vi "PiecesMovement.vi"(8 "Move to":i32[](array[numeric]), 9 "Move from":i32[](array[numeric]), 10 "Turn":T1, 11 "Input Squares":T2[][](array[typedef])) -> (0 "Short Castle?":bool, 1 "Beat in the Passage?":bool, 2 "Last Square?":bool, 3 "Possible Move?":bool, 4 "Long Castle?":bool, 5 "Possible Moves":bool[][](array[boolean]))   [LabVIEW 2019]
doc: "This VI checks if movement of the piece is executed properly"
uses:
  #typedef_SquareType.ctl
  #typedef_Color.ctl
  #typedef_Piece.ctl
  #typedef_PieceType.ctl
panel:
  out "?":u16[][](array[ring])
  out "Last Square":bool[][](array[boolean])
  out "Beat in the Passage":bool[][](array[boolean])
  out "Short Castle":bool[][](array[boolean])
  out "Long Castle":bool[][](array[boolean])
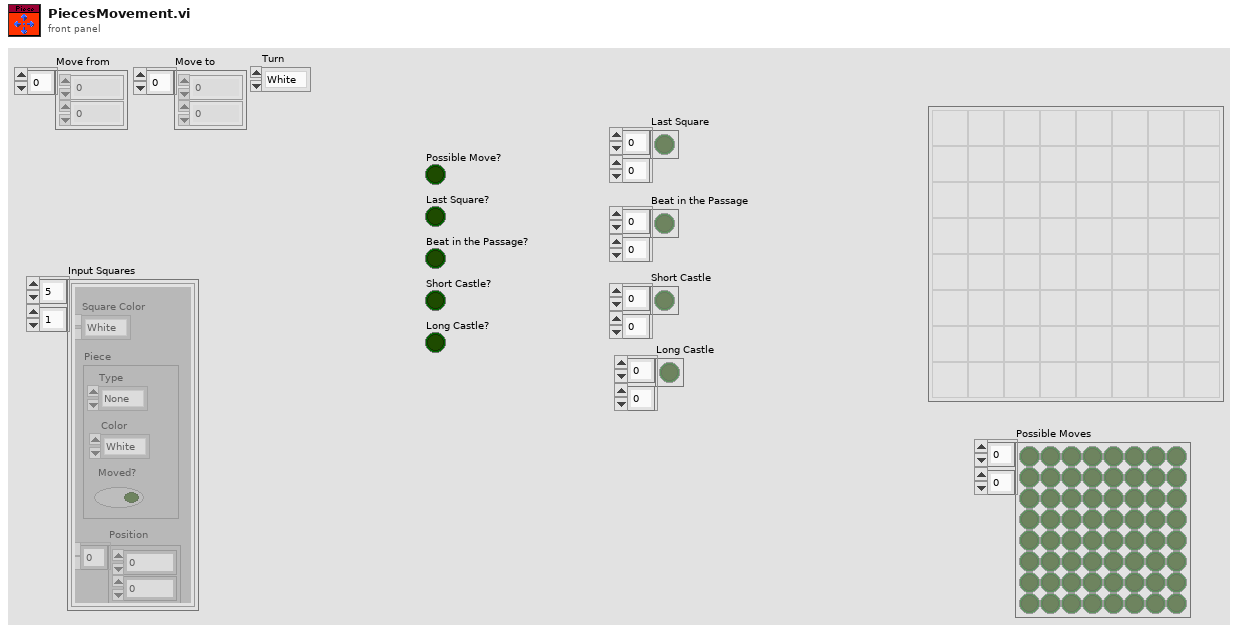
[diagram p1: front panel]
types:
  T1 = typedef "#typedef_Color.ctl" = enum16{"White", "Black"}
  T2 = typedef "#typedef_SquareType.ctl" = cluster{"Square Color":T1, "Position":i32[], "Piece":T3}
  T3 = typedef "#typedef_Piece.ctl" = cluster{"Type":T4, "Color":T1, "Moved?":bool}
  T4 = typedef "#typedef_PieceType.ctl" = enum16{"None", "Pawn", "Knight", "Bishop", "Rook", "Queen", "King"}
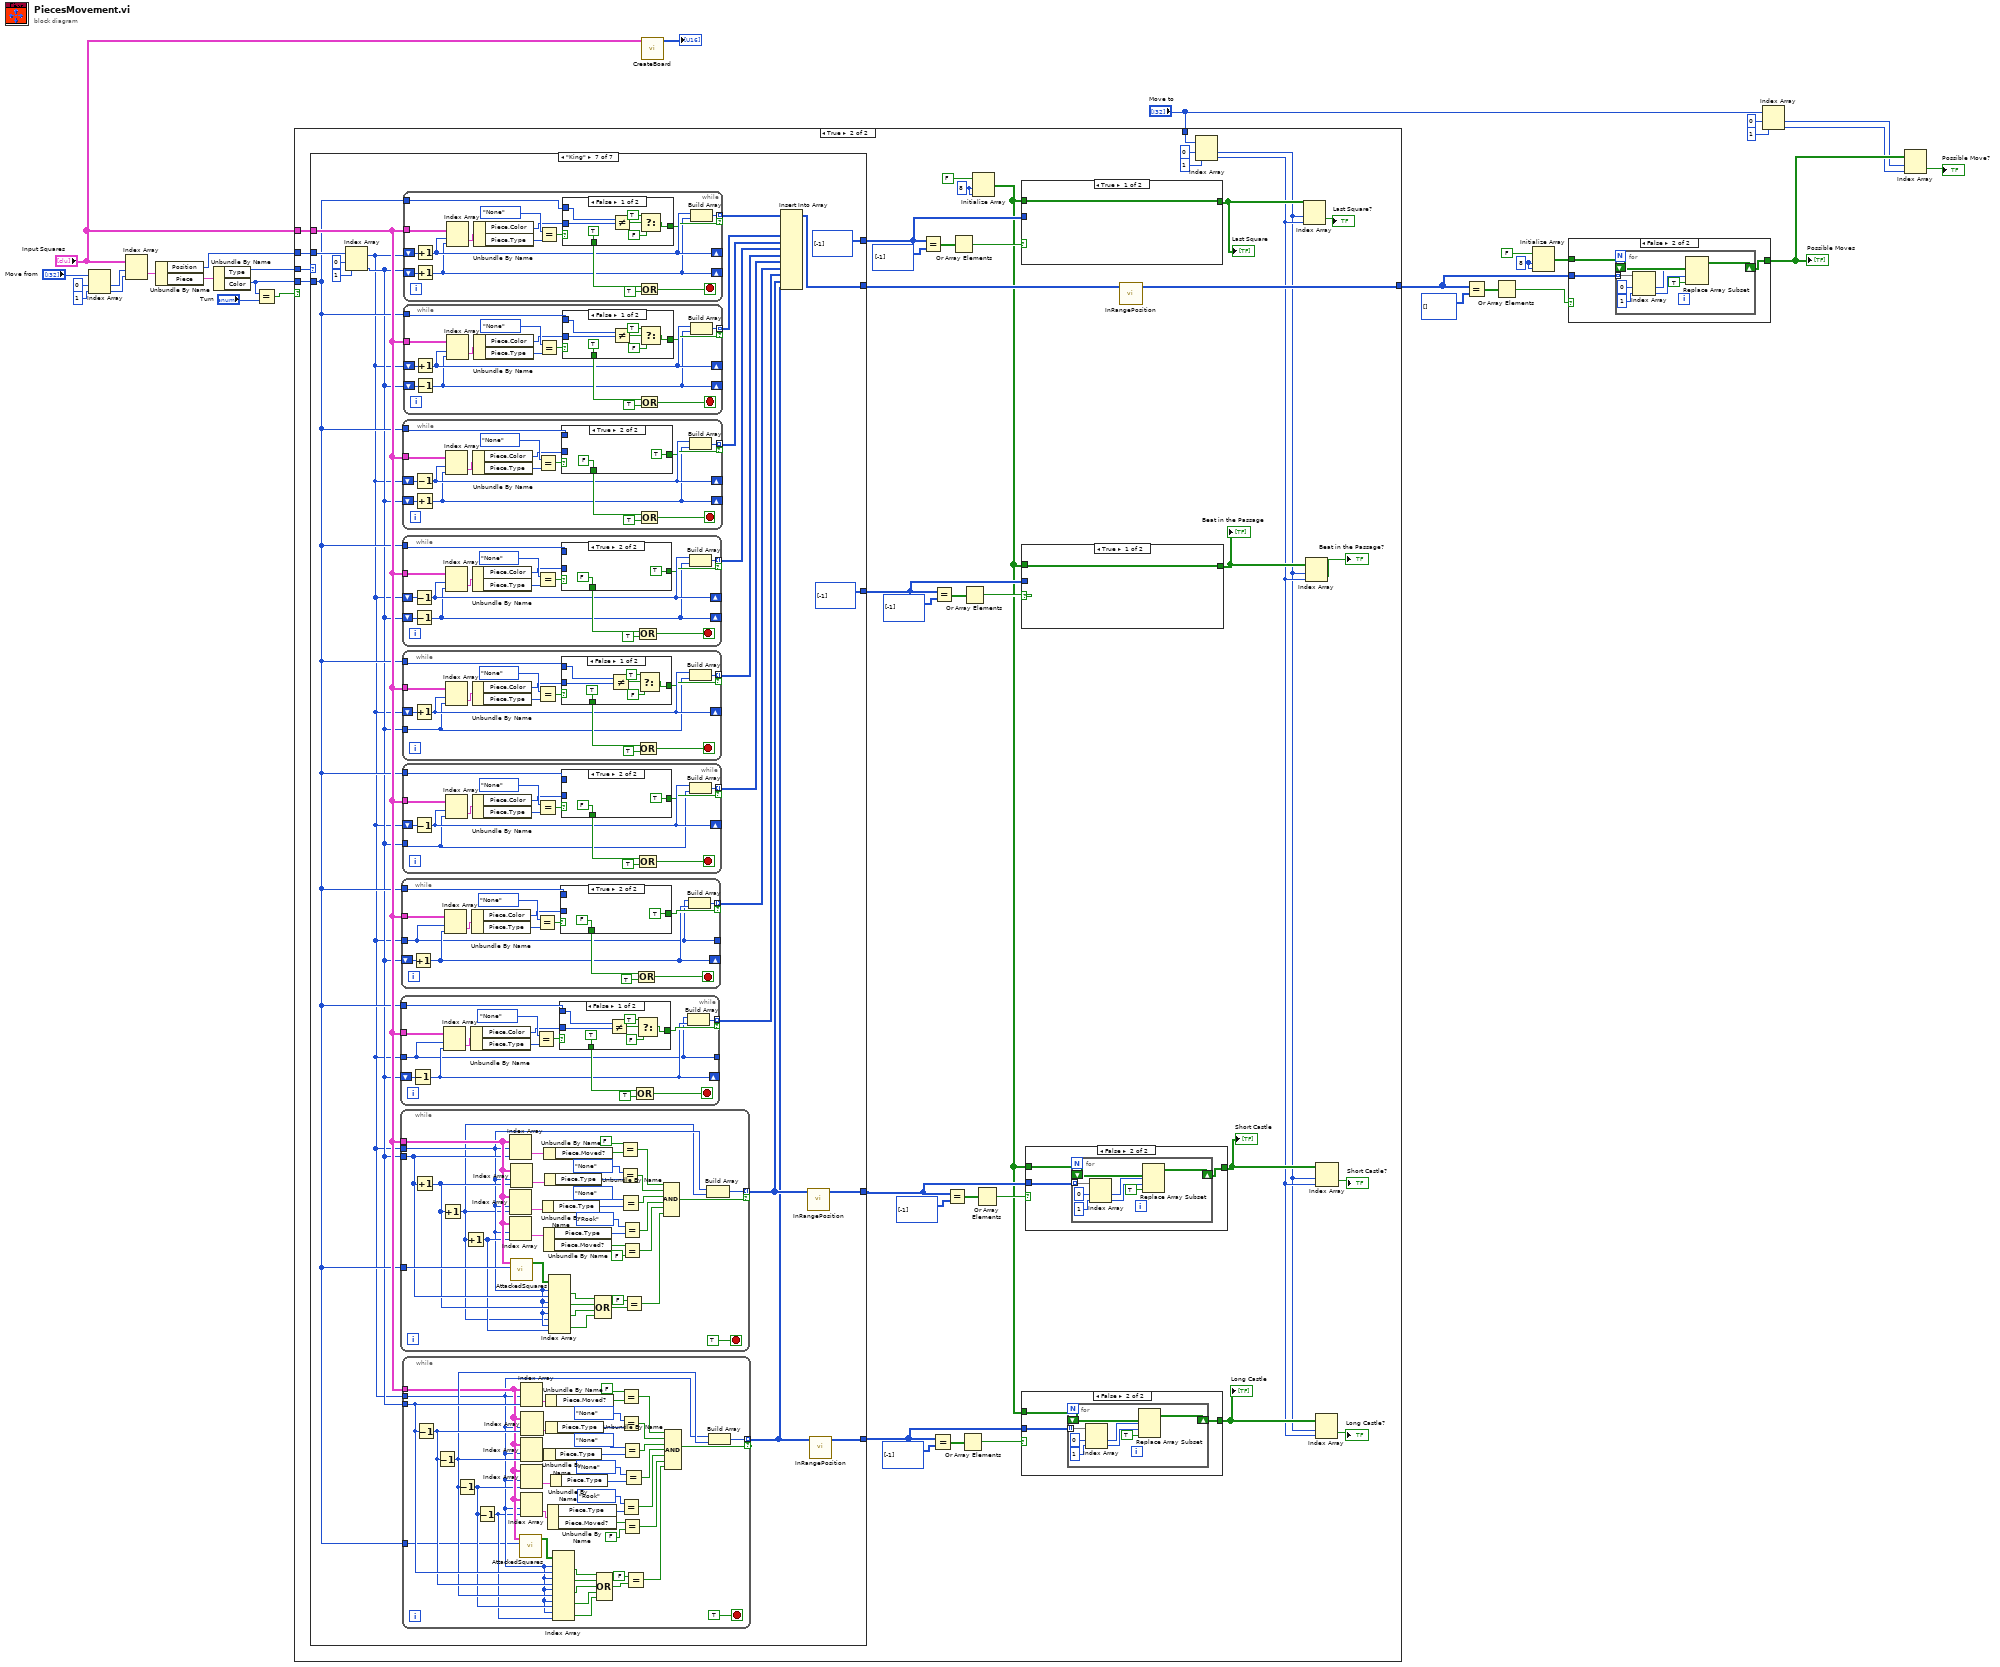
[diagram p0: block diagram]
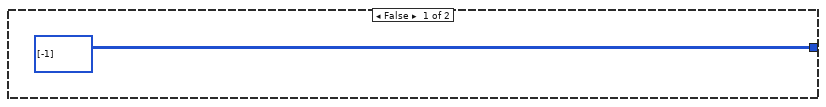
[diagram p3: hidden frame]
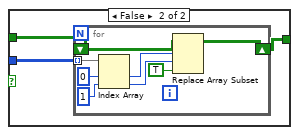
[diagram p6: hidden frame]
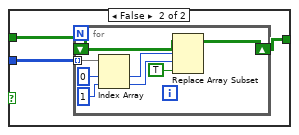
[diagram p7: hidden frame]
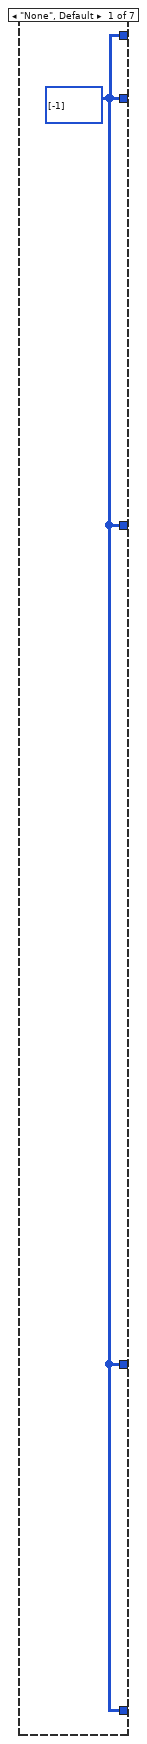
[diagram p8: hidden frame]
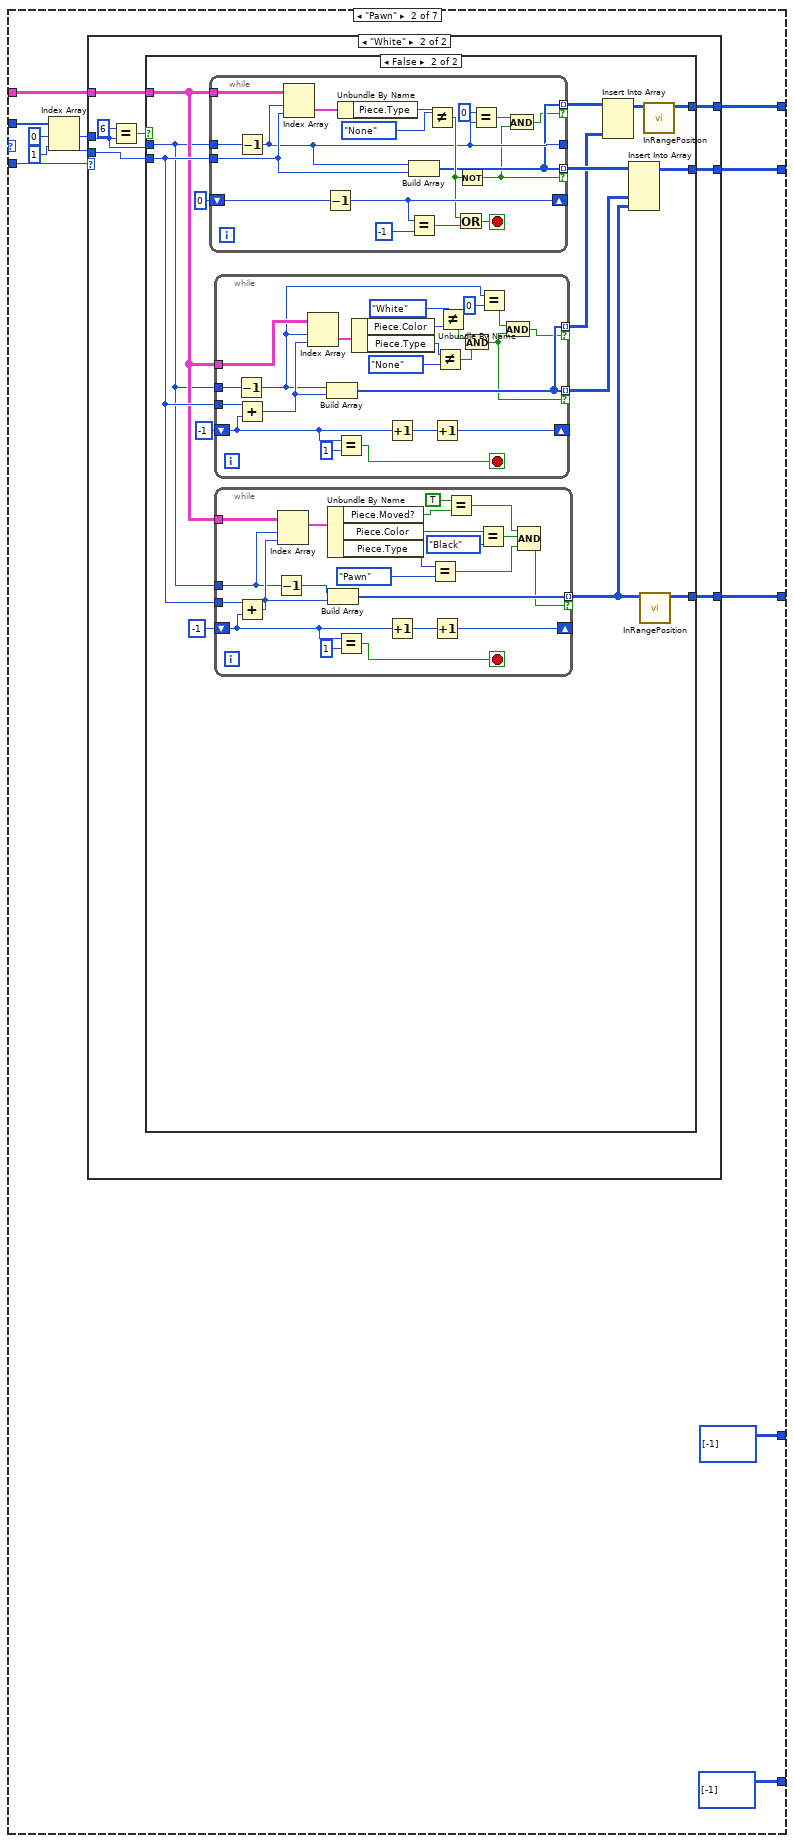
[diagram p9: hidden frame]
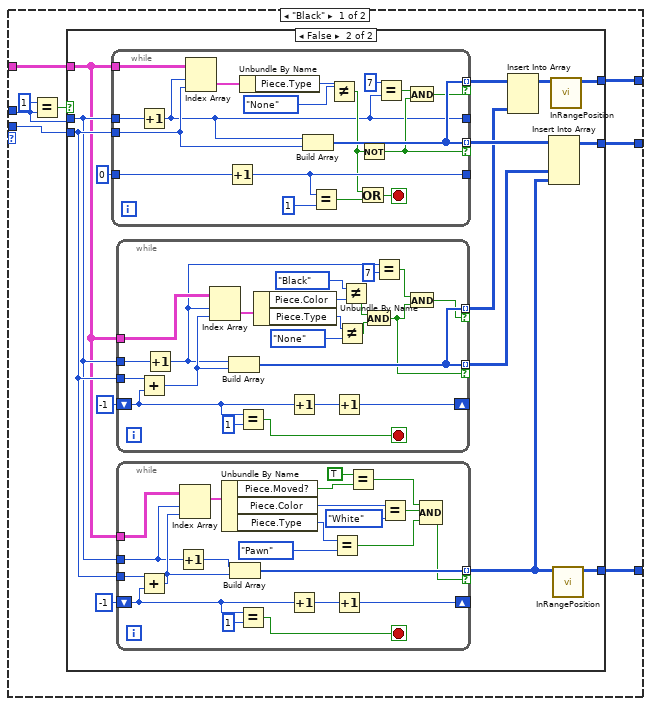
[diagram p10: hidden frame]
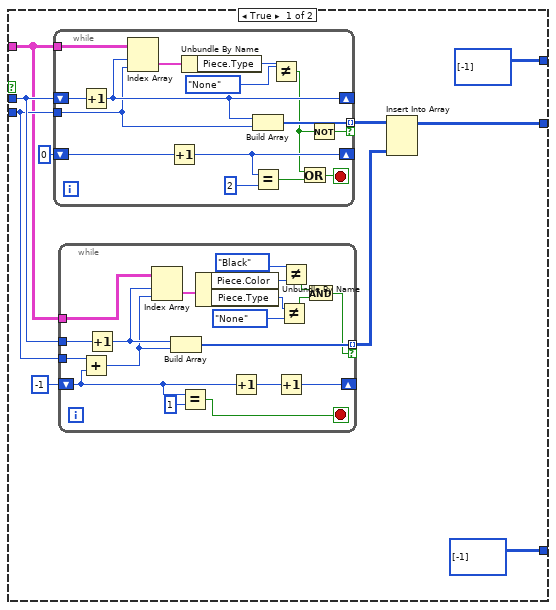
[diagram p11: hidden frame]
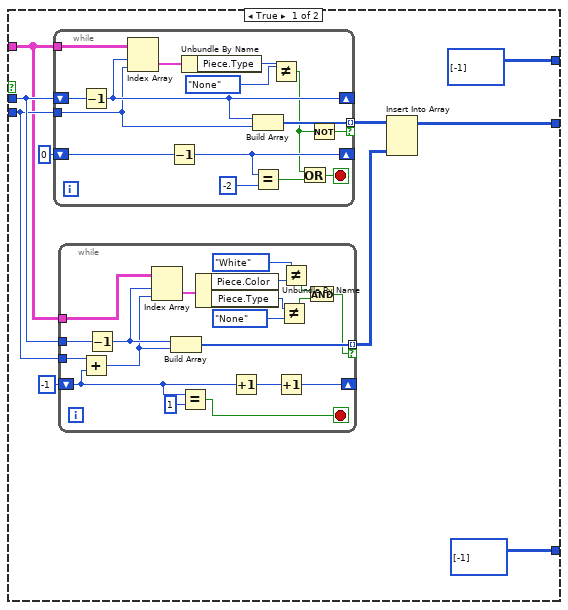
[diagram p12: hidden frame]
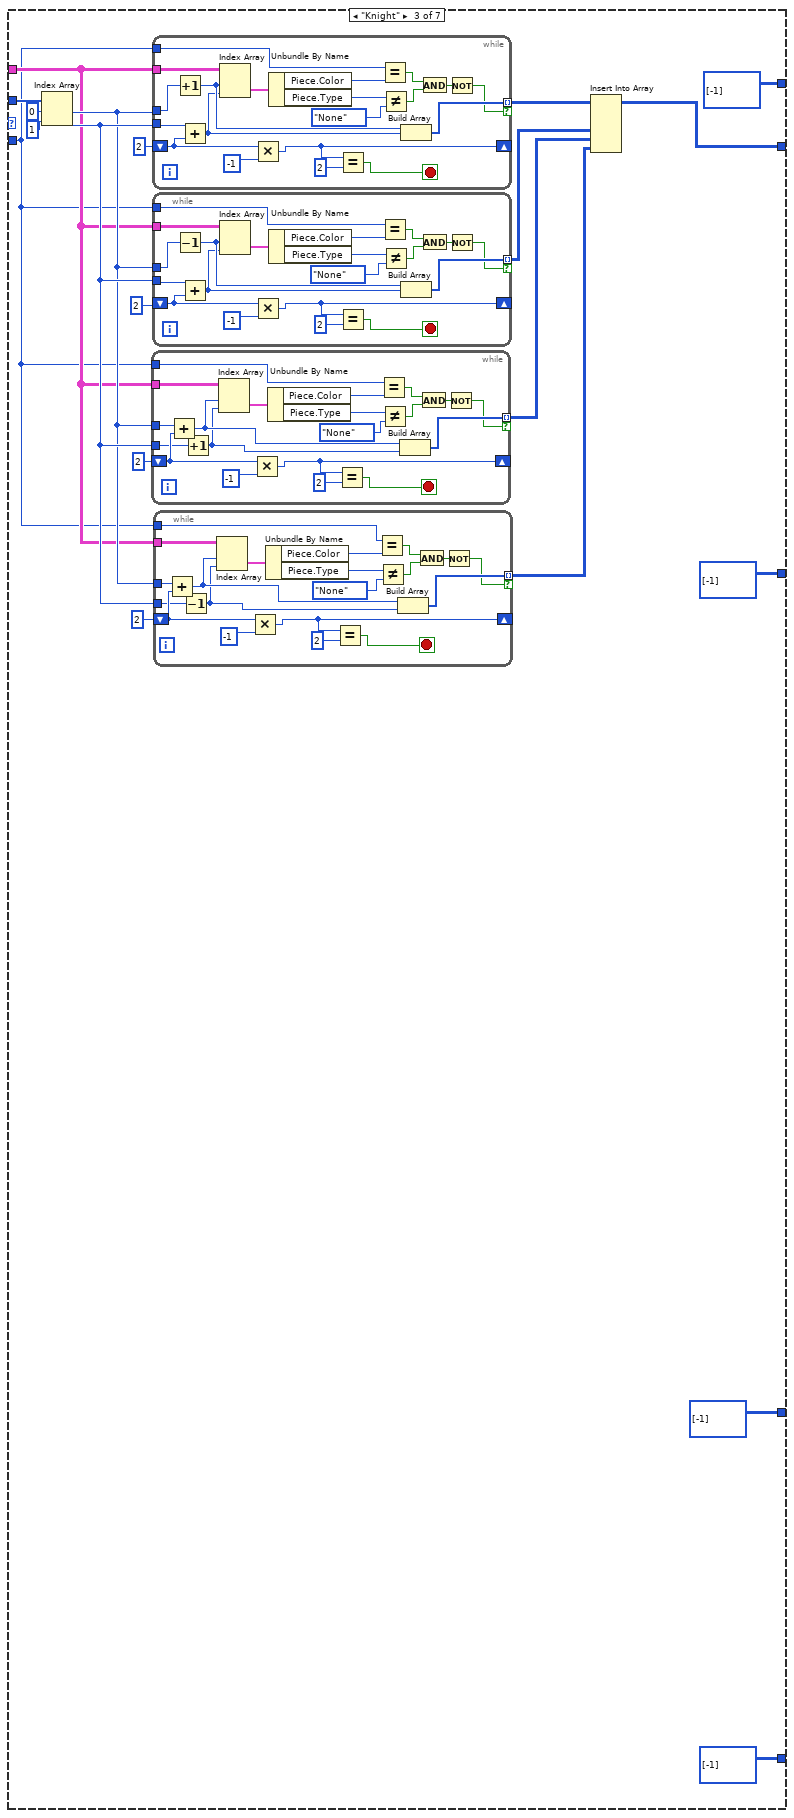
[diagram p13: hidden frame]
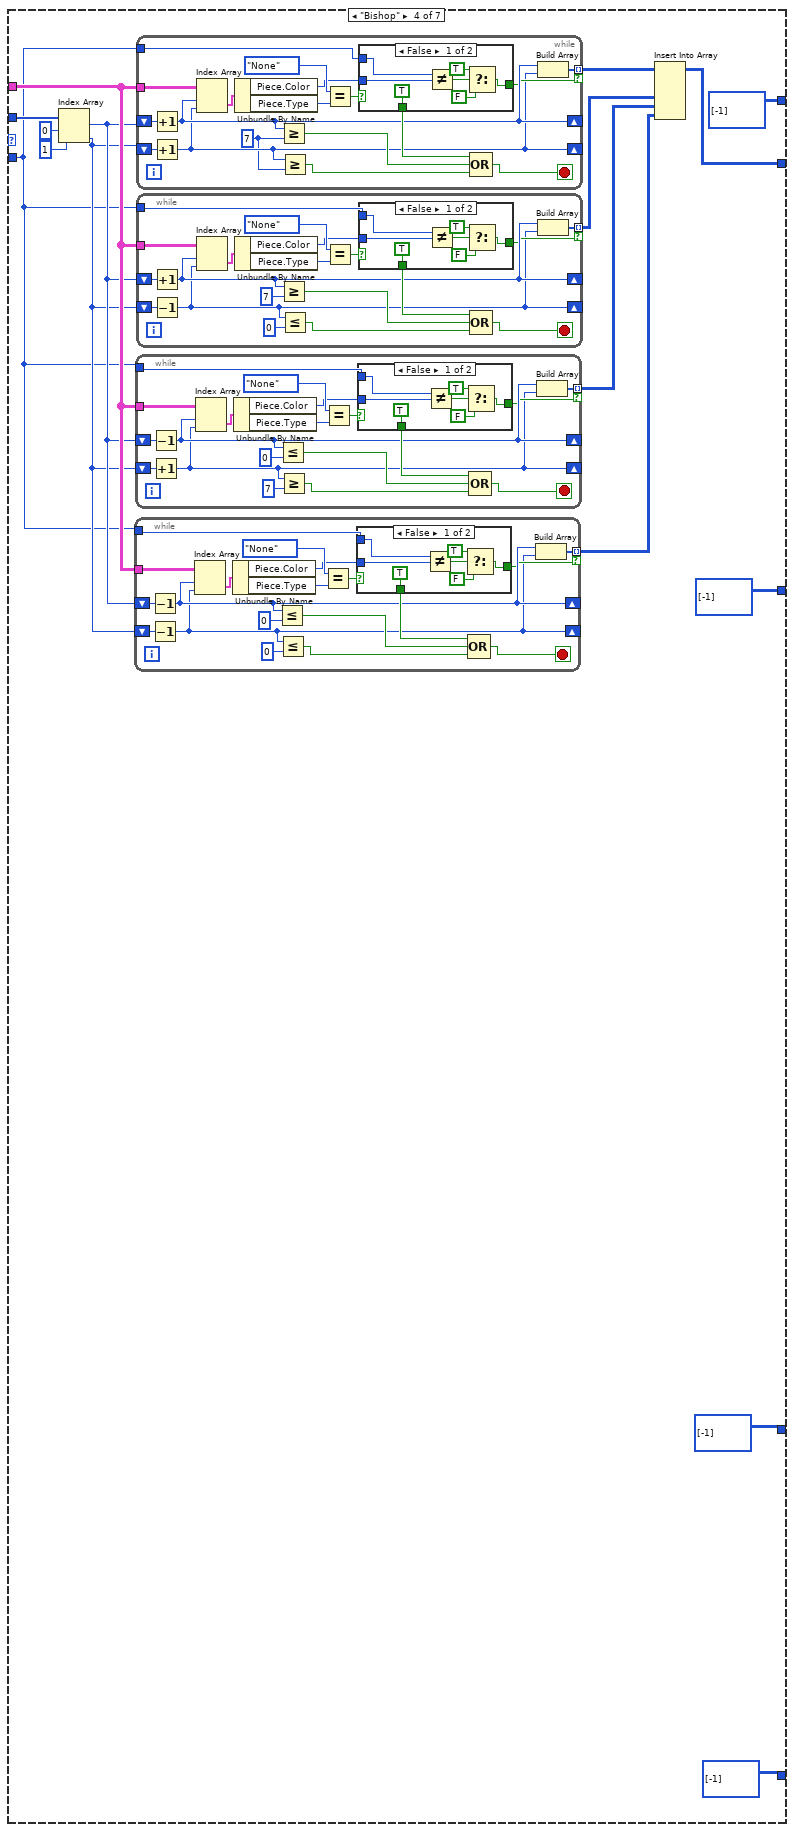
[diagram p14: hidden frame]
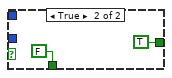
[diagram p15: hidden frame]
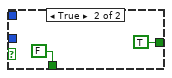
[diagram p16: hidden frame]
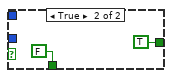
[diagram p17: hidden frame]
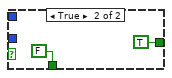
[diagram p18: hidden frame]
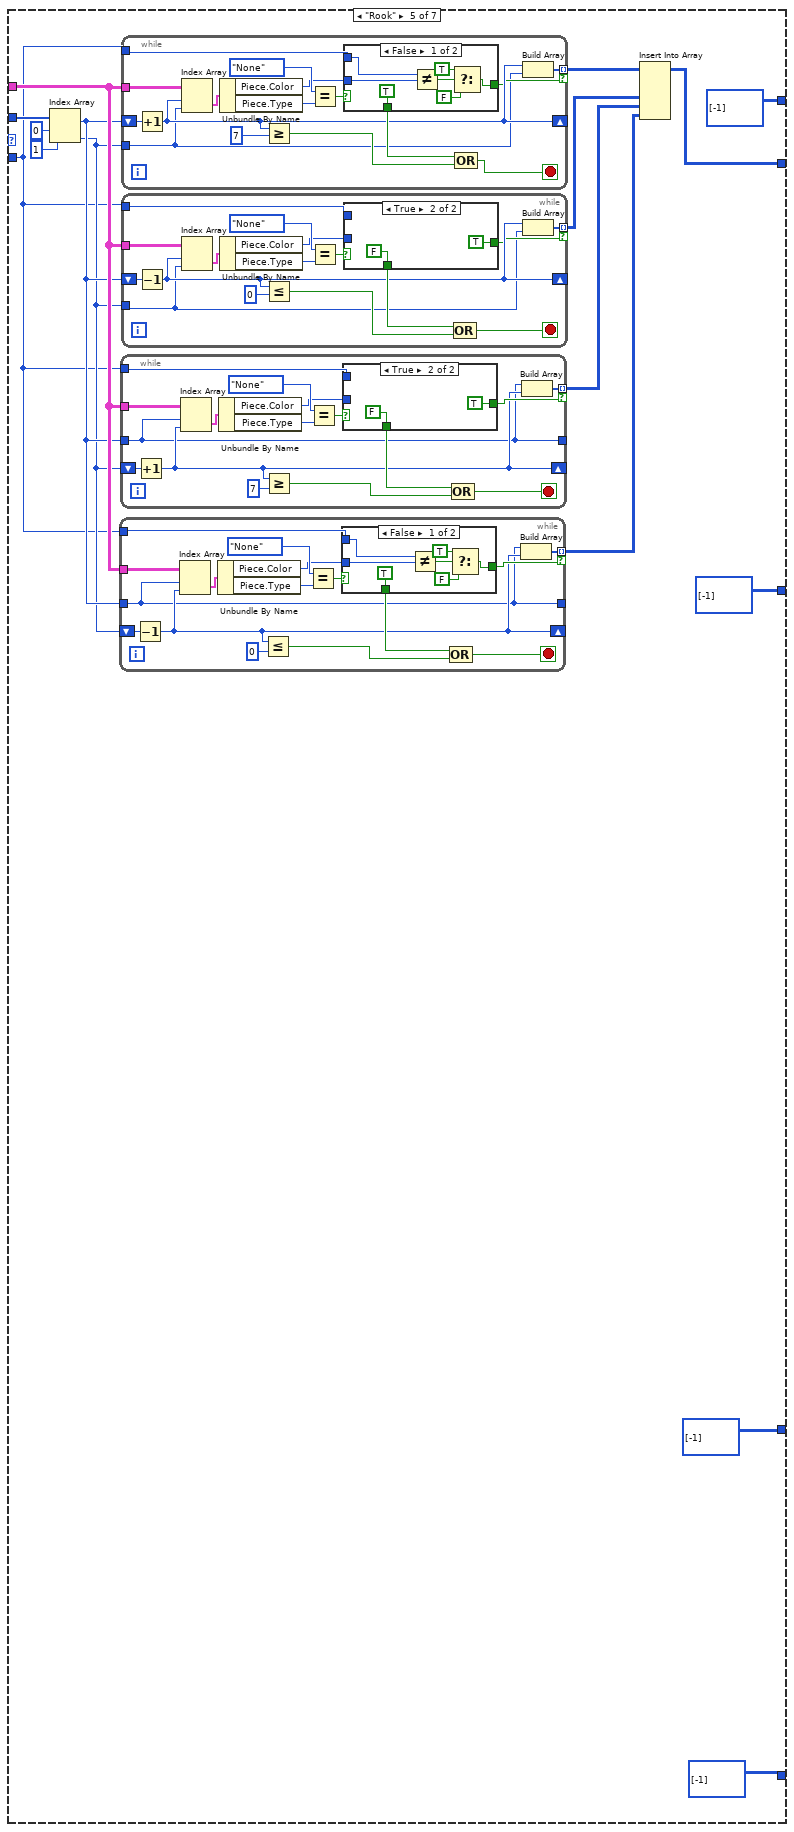
[diagram p19: hidden frame]
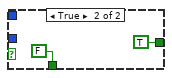
[diagram p20: hidden frame]
diagram:
  w15 = 8 ("dimension size")
  n1 = Index Array(array="Move from", index #1=0 ("index"), index #2=1 ("index")) -> (element #1=w25:i32, element #2=w26:i32)
  n2 = Index Array(array="Input Squares", index (row)=w25, index (col)=w26) -> (element=w27:T2)
  n3 = Unbundle By Name(w27) -> ("Position"=w22:i32[], "Piece"=w28:T3)
  n4 = Unbundle By Name(w28) -> ("Type"=w21:T4, "Color"=w20:T1)
  n5 = Equal?(x=w20, y="Turn") -> (x = y?=w19:bool)
  n6 = case shown="True" w19 {
    tunnel: w21 -> [_ w67]
    tunnel: w22 -> [_ w66]
    tunnel: w20 -> [_ w65]
    tunnel: "Input Squares" -> [_ w64]
    tunnel: [i32[][] [[-1]] w32] -> w16
    tunnel: "Move to" -> [_ w41]
    frame False {
    }
    frame True {
      w62 = 8 ("dimension size")
      n7 = case shown="\"King\"" w67 {
        tunnel: w66 -> [_ w125 w393 w500 w627 w747 w980]
        tunnel: w65 -> [_ w128 w392 w492 w619 w739 w968]
        tunnel: w64 -> [_ w122 w394 w495 w622 w742 w969]
        tunnel: [w116 w121 w391 w491 w618 w734 w972] -> w63
        tunnel: [w116 w120 i32[][] [[-1]] i32[][] [[-1]] i32[][] [[-1]] i32[][] [[-1]] i32[][] [[-1]]] -> w58
        tunnel: [w116 w119 i32[][] [[-1]] i32[][] [[-1]] i32[][] [[-1]] i32[][] [[-1]] i32[][] [[-1]]] -> w54
        tunnel: [w116 i32[][] [[-1]] i32[][] [[-1]] i32[][] [[-1]] i32[][] [[-1]] i32[][] [[-1]] w963] -> w49
        tunnel: [w116 i32[][] [[-1]] i32[][] [[-1]] i32[][] [[-1]] i32[][] [[-1]] i32[][] [[-1]] w962] -> w45
        frame "None", Default {
          w116 = i32[][] [[-1]]
        }
        frame "Pawn" {
          n8 = Index Array(array=w125, index #1=0 ("index"), index #2=1 ("index")) -> (element #1=w124:i32, element #2=w123:i32)
          n9 = case shown="\"White\"" w128 {
            tunnel: w124 -> [w132 w261]
            tunnel: w123 -> [w133 w262]
            tunnel: w122 -> [w134 w263]
            tunnel: [w131 w260] -> w121
            tunnel: [w130 w259] -> w119
            tunnel: [w129 w258] -> w120
            frame "Black" {
              n10 = Equal?(x=1, y=w132) -> (x = y?=w135:bool)
              n11 = case shown="False" w135 {
                tunnel: w134 -> [w142 w187]
                tunnel: w133 -> [w143 w189]
                tunnel: w132 -> [w144 w188]
                tunnel: [w139 w191] -> w131
                tunnel: [i32[][] [[-1]] w181] -> w130
                tunnel: [i32[][] [[-1]] w182] -> w129
                frame True {
                  n12 = while {
                    tunnel: w142 -> [w180]
                    tunnel: w143 -> [w170]
                    shift-right: [w171] -> _
                    shift-left: w144 -> [w179]
                    tunnel: [w169] -> w141 mode=indexing if=w166
                    shift-right: [w173] -> _
                    shift-left: 0 -> [w178]
                    stop <- w168 stop-if-true
                    n13 = Increment(x=w179) -> (x+1=w171:i32)
                    n14 = Index Array(array=w180, index (row)=w171, index (col)=w170) -> (element=w177:T2)
                    n15 = Increment(x=w178) -> (x+1=w173:i32)
                    n16 = Unbundle By Name(w177) -> ("Piece.Type"=w176:T4)
                    n17 = Build Array(w171, w170) -> (w169:i32[])
                    n18 = Equal?(x=w173, y=2 ("x")) -> (x = y?=w174:bool)
                    n19 = Not Equal?(x=#typedef_PieceType."None" ("y"), y=w176) -> (x != y?=w167:bool)
                    n20 = Or(x=w167, y=w174) -> (x .or. y?=w168:bool)
                    n21 = Not(x=w167) -> (.not. x?=w166:bool)
                  }
                  n22 = while {
                    tunnel: w144 -> [w161]
                    tunnel: w143 -> [w160]
                    tunnel: w142 -> [w158]
                    tunnel: [w152] -> w140 mode=indexing if=w147
                    shift-right: [w164] -> _
                    shift-left: -1 -> [w159]
                    stop <- w162 stop-if-true
                    n23 = Add(x=w160, y=w159) -> (x+y=w153:i32)
                    n24 = Increment(x=w161) -> (x+1=w154:i32)
                    n25 = Index Array(array=w158, index (row)=w154, index (col)=w153) -> (element=w157:T2)
                    n26 = Build Array(w154, w153) -> (w152:i32[])
                    n27 = Equal?(x=w159, y=1) -> (x = y?=w162:bool)
                    n28 = Unbundle By Name(w157) -> ("Piece.Color"=w151:T1, "Piece.Type"=w156:T4)
                    n29 = Increment(x=w159) -> (x+1=w165:i32)
                    n30 = Increment(x=w165) -> (x+1=w164:i32)
                    n31 = Not Equal?(x=w156, y=#typedef_PieceType."None") -> (x != y?=w149:bool)
                    n32 = Not Equal?(x=#typedef_Color."Black", y=w151) -> (x != y?=w148:bool)
                    n33 = And(x=w148, y=w149) -> (x .and. y?=w147:bool)
                  }
                  n34 = Insert Into Array(array=w141, new element=w140) -> (w139:i32[][])  [unwired: 2 in]
                }
                frame False {
                  n35 = while {
                    tunnel: w187 -> [w257]
                    tunnel: w189 -> [w248]
                    tunnel: 0 -> [w255]
                    tunnel: [w250] -> _
                    tunnel: [w246] -> w193 mode=indexing if=w244
                    tunnel: w188 -> [w256]
                    tunnel: [w241] -> _
                    tunnel: [w246] -> w184 mode=indexing if=w243
                    stop <- w247 stop-if-true
                    n36 = Increment(x=w256) -> (x+1=w241:i32)
                    n37 = Index Array(array=w257, index (row)=w241, index (col)=w248) -> (element=w254:T2)
                    n38 = Increment(x=w255) -> (x+1=w250:i32)
                    n39 = Unbundle By Name(w254) -> ("Piece.Type"=w253:T4)
                    n40 = Build Array(w241, w248) -> (w246:i32[])
                    n41 = Equal?(x=w250, y=1 ("x")) -> (x = y?=w251:bool)
                    n42 = Not Equal?(x=#typedef_PieceType."None" ("y"), y=w253) -> (x != y?=w245:bool)
                    n43 = Or(x=w245, y=w251) -> (x .or. y?=w247:bool)
                    n44 = Not(x=w245) -> (.not. x?=w244:bool)
                    n45 = Equal?(x=7, y=w241) -> (x = y?=w242:bool)
                    n46 = And(x=w242, y=w244) -> (x .and. y?=w243:bool)
                  }
                  n47 = while {
                    tunnel: w188 -> [w235]
                    tunnel: w189 -> [w234]
                    tunnel: w187 -> [w232]
                    tunnel: [w223] -> w192 mode=indexing if=w222
                    shift-right: [w238] -> _
                    shift-left: -1 -> [w233]
                    tunnel: [w223] -> w183 mode=indexing if=w218
                    stop <- w236 stop-if-true
                    n48 = Add(x=w234, y=w233) -> (x+y=w228:i32)
                    n49 = Increment(x=w235) -> (x+1=w220:i32)
                    n50 = Index Array(array=w232, index (row)=w220, index (col)=w228) -> (element=w231:T2)
                    n51 = Build Array(w220, w228) -> (w223:i32[])
                    n52 = Equal?(x=w233, y=1) -> (x = y?=w236:bool)
                    n53 = Unbundle By Name(w231) -> ("Piece.Color"=w227:T1, "Piece.Type"=w230:T4)
                    n54 = Increment(x=w233) -> (x+1=w239:i32)
                    n55 = Increment(x=w239) -> (x+1=w238:i32)
                    n56 = Not Equal?(x=w230, y=#typedef_PieceType."None") -> (x != y?=w224:bool)
                    n57 = Not Equal?(x=#typedef_Color."Black", y=w227) -> (x != y?=w225:bool)
                    n58 = And(x=w225, y=w224) -> (x .and. y?=w222:bool)
                    n59 = Equal?(x=w220, y=7) -> (x = y?=w221:bool)
                    n60 = And(x=w221, y=w222) -> (x .and. y?=w218:bool)
                  }
                  n61 = while {
                    tunnel: w188 -> [w207]
                    tunnel: w189 -> [w213]
                    tunnel: w187 -> [w211]
                    tunnel: [w208] -> w186 mode=indexing if=w197
                    shift-right: [w216] -> _
                    shift-left: -1 -> [w212]
                    stop <- w214 stop-if-true
                    n62 = Add(x=w213, y=w212) -> (x+y=w209:i32)
                    n63 = Increment(x=w207) -> (x+1=w196:i32)
                    n64 = Index Array(array=w211, index (row)=w207, index (col)=w209) -> (element=w210:T2)
                    n65 = Unbundle By Name(w210) -> ("Piece.Moved?"=w203:bool, "Piece.Color"=w206:T1, "Piece.Type"=w205:T4)
                    n66 = Build Array(w196, w209) -> (w208:i32[])
                    n67 = Equal?(x=w212, y=1) -> (x = y?=w214:bool)
                    n68 = Increment(x=w212) -> (x+1=w217:i32)
                    n69 = Equal?(x=w205, y=#typedef_PieceType."Pawn") -> (x = y?=w199:bool)
                    n70 = Increment(x=w217) -> (x+1=w216:i32)
                    n71 = Equal?(x=TRUE, y=w203) -> (x = y?=w198:bool)
                    n72 = Equal?(x=w206, y=#typedef_Color."White" ("x")) -> (x = y?=w200:bool)
                    n73 = Compound Arithmetic op=AND(w198, w200, w199) -> (w197:bool)
                  }
                  n74 = Insert Into Array(array=w184, new element=w183) -> (w185:i32[][])  [unwired: 2 in]
                  n75 = Insert Into Array(array=w193, new element #1=w192, new element #2=w186) -> (w191:i32[][])  [unwired: 2 in]
                  n76 = call "InRangePosition.vi"("Input Positions in"=w185) -> ("Output Positions"=w182:i32[][])  [unwired: 10 in]
                  n77 = call "InRangePosition.vi"("Input Positions in"=w186) -> ("Output Positions"=w181:i32[][])  [unwired: 10 in]
                }
              }
            }
            frame "White" {
              n78 = Equal?(x=6, y=w261) -> (x = y?=w264:bool)
              n79 = case shown="False" w264 {
                tunnel: w263 -> [w271 w318]
                tunnel: w262 -> [w272 w319]
                tunnel: w261 -> [w273 w315]
                tunnel: [w268 w320] -> w260
                tunnel: [i32[][] [[-1]] w310] -> w259
                tunnel: [i32[][] [[-1]] w311] -> w258
                frame True {
                  n80 = while {
                    tunnel: w271 -> [w309]
                    tunnel: w272 -> [w299]
                    shift-right: [w300] -> _
                    shift-left: w273 -> [w308]
                    tunnel: [w298] -> w270 mode=indexing if=w295
                    shift-right: [w302] -> _
                    shift-left: 0 -> [w307]
                    stop <- w297 stop-if-true
                    n81 = Decrement(x=w308) -> (x-1=w300:i32)
                    n82 = Index Array(array=w309, index (row)=w300, index (col)=w299) -> (element=w306:T2)
                    n83 = Decrement(x=w307) -> (x-1=w302:i32)
                    n84 = Unbundle By Name(w306) -> ("Piece.Type"=w305:T4)
                    n85 = Build Array(w300, w299) -> (w298:i32[])
                    n86 = Equal?(x=w302, y=-2 ("x")) -> (x = y?=w303:bool)
                    n87 = Not Equal?(x=#typedef_PieceType."None" ("y"), y=w305) -> (x != y?=w296:bool)
                    n88 = Or(x=w296, y=w303) -> (x .or. y?=w297:bool)
                    n89 = Not(x=w296) -> (.not. x?=w295:bool)
                  }
                  n90 = while {
                    tunnel: w273 -> [w290]
                    tunnel: w272 -> [w289]
                    tunnel: w271 -> [w287]
                    tunnel: [w281] -> w269 mode=indexing if=w276
                    shift-right: [w293] -> _
                    shift-left: -1 -> [w288]
                    stop <- w291 stop-if-true
                    n91 = Add(x=w289, y=w288) -> (x+y=w282:i32)
                    n92 = Decrement(x=w290) -> (x-1=w283:i32)
                    n93 = Index Array(array=w287, index (row)=w283, index (col)=w282) -> (element=w286:T2)
                    n94 = Build Array(w283, w282) -> (w281:i32[])
                    n95 = Equal?(x=w288, y=1) -> (x = y?=w291:bool)
                    n96 = Unbundle By Name(w286) -> ("Piece.Color"=w280:T1, "Piece.Type"=w285:T4)
                    n97 = Increment(x=w288) -> (x+1=w294:i32)
                    n98 = Increment(x=w294) -> (x+1=w293:i32)
                    n99 = Not Equal?(x=w285, y=#typedef_PieceType."None") -> (x != y?=w278:bool)
                    n100 = Not Equal?(x=#typedef_Color."White", y=w280) -> (x != y?=w277:bool)
                    n101 = And(x=w277, y=w278) -> (x .and. y?=w276:bool)
                  }
                  n102 = Insert Into Array(array=w270, new element=w269) -> (w268:i32[][])  [unwired: 2 in]
                }
                frame False {
                  n103 = while {
                    tunnel: w318 -> [w386]
                    tunnel: w319 -> [w377]
                    tunnel: [w372] -> w322 mode=indexing if=w370
                    shift-right: [w379] -> _
                    shift-left: 0 -> [w384]
                    tunnel: [w372] -> w314 mode=indexing if=w369
                    tunnel: w315 -> [w385]
                    tunnel: [w374] -> _
                    stop <- w376 stop-if-true
                    n104 = Decrement(x=w385) -> (x-1=w374:i32)
                    n105 = Index Array(array=w386, index (row)=w374, index (col)=w377) -> (element=w383:T2)
                    n106 = Decrement(x=w384) -> (x-1=w379:i32)
                    n107 = Unbundle By Name(w383) -> ("Piece.Type"=w382:T4)
                    n108 = Build Array(w374, w377) -> (w372:i32[])
                    n109 = Equal?(x=w379, y=-1 ("x")) -> (x = y?=w380:bool)
                    n110 = Not Equal?(x=#typedef_PieceType."None" ("y"), y=w382) -> (x != y?=w375:bool)
                    n111 = Or(x=w375, y=w380) -> (x .or. y?=w376:bool)
                    n112 = Not(x=w375) -> (.not. x?=w370:bool)
                    n113 = Equal?(x=0, y=w374) -> (x = y?=w371:bool)
                    n114 = And(x=w371, y=w370) -> (x .and. y?=w369:bool)
                  }
                  n115 = while {
                    tunnel: w315 -> [w364]
                    tunnel: w319 -> [w363]
                    tunnel: w318 -> [w361]
                    tunnel: [w352] -> w321 mode=indexing if=w348
                    shift-right: [w367] -> _
                    shift-left: -1 -> [w362]
                    tunnel: [w352] -> w313 mode=indexing if=w347
                    stop <- w365 stop-if-true
                    n116 = Decrement(x=w364) -> (x-1=w350:i32)
                    n117 = Add(x=w363, y=w362) -> (x+y=w357:i32)
                    n118 = Index Array(array=w361, index (row)=w350, index (col)=w357) -> (element=w360:T2)
                    n119 = Build Array(w350, w357) -> (w352:i32[])
                    n120 = Equal?(x=w362, y=1) -> (x = y?=w365:bool)
                    n121 = Unbundle By Name(w360) -> ("Piece.Color"=w356:T1, "Piece.Type"=w359:T4)
                    n122 = Increment(x=w362) -> (x+1=w368:i32)
                    n123 = Increment(x=w368) -> (x+1=w367:i32)
                    n124 = Not Equal?(x=w359, y=#typedef_PieceType."None") -> (x != y?=w354:bool)
                    n125 = Not Equal?(x=#typedef_Color."White", y=w356) -> (x != y?=w353:bool)
                    n126 = And(x=w353, y=w354) -> (x .and. y?=w348:bool)
                    n127 = Equal?(x=w350, y=0 ("x")) -> (x = y?=w349:bool)
                    n128 = And(x=w349, y=w348) -> (x .and. y?=w347:bool)
                  }
                  n129 = while {
                    tunnel: w315 -> [w336]
                    tunnel: w319 -> [w342]
                    tunnel: w318 -> [w340]
                    tunnel: [w337] -> w316 mode=indexing if=w326
                    shift-right: [w345] -> _
                    shift-left: -1 -> [w341]
                    stop <- w343 stop-if-true
                    n130 = Add(x=w342, y=w341) -> (x+y=w338:i32)
                    n131 = Decrement(x=w336) -> (x-1=w325:i32)
                    n132 = Index Array(array=w340, index (row)=w336, index (col)=w338) -> (element=w339:T2)
                    n133 = Unbundle By Name(w339) -> ("Piece.Moved?"=w332:bool, "Piece.Color"=w335:T1, "Piece.Type"=w334:T4)
                    n134 = Build Array(w325, w338) -> (w337:i32[])
                    n135 = Equal?(x=w341, y=1) -> (x = y?=w343:bool)
                    n136 = Increment(x=w341) -> (x+1=w346:i32)
                    n137 = Equal?(x=w334, y=#typedef_PieceType."Pawn") -> (x = y?=w328:bool)
                    n138 = Increment(x=w346) -> (x+1=w345:i32)
                    n139 = Equal?(x=TRUE, y=w332) -> (x = y?=w327:bool)
                    n140 = Equal?(x=w335, y=#typedef_Color."Black" ("x")) -> (x = y?=w329:bool)
                    n141 = Compound Arithmetic op=AND(w327, w329, w328) -> (w326:bool)
                  }
                  n142 = Insert Into Array(array=w314, new element=w313) -> (w312:i32[][])  [unwired: 2 in]
                  n143 = Insert Into Array(array=w322, new element #1=w321, new element #2=w316) -> (w320:i32[][])  [unwired: 2 in]
                  n144 = call "InRangePosition.vi"("Input Positions in"=w316) -> ("Output Positions"=w310:i32[][])  [unwired: 10 in]
                  n145 = call "InRangePosition.vi"("Input Positions in"=w312) -> ("Output Positions"=w311:i32[][])  [unwired: 10 in]
                }
              }
            }
          }
        }
        frame "Knight" {
          n146 = Index Array(array=w393, index #1=0 ("index"), index #2=1 ("index")) -> (element #1=w399:i32, element #2=w400:i32)
          n147 = while {
            tunnel: w394 -> [w446]
            tunnel: w399 -> [w433]
            tunnel: w400 -> [w431]
            shift-right: [w439] -> _
            shift-left: 2 -> [w432]
            tunnel: [w436] -> w396 mode=indexing if=w434
            tunnel: w392 -> [w427]
            stop <- w437 stop-if-true
            n148 = Add(x=w433, y=w432) -> (x+y=w430:i32)
            n149 = Increment(x=w431) -> (x+1=w429:i32)
            n150 = Index Array(array=w446, index (row)=w430, index (col)=w429) -> (element=w444:T2)
            n151 = Multiply(x=w432, y=-1) -> (x*y=w439:i32)
            n152 = Unbundle By Name(w444) -> ("Piece.Color"=w443:T1, "Piece.Type"=w442:T4)
            n153 = Equal?(x=w439, y=2) -> (x = y?=w437:bool)
            n154 = Equal?(x=w427, y=w443) -> (x = y?=w441:bool)
            n155 = Not Equal?(x=w442, y=#typedef_PieceType."None") -> (x != y?=w440:bool)
            n156 = Build Array(w430, w429) -> (w436:i32[])
            n157 = And(x=w441, y=w440) -> (x .and. y?=w435:bool)
            n158 = Not(x=w435) -> (.not. x?=w434:bool)
          }
          n159 = while {
            tunnel: w394 -> [w486]
            tunnel: w399 -> [w482]
            tunnel: w400 -> [w483]
            shift-right: [w476] -> _
            shift-left: 2 -> [w484]
            tunnel: [w471] -> w398 mode=indexing if=w469
            tunnel: w392 -> [w467]
            stop <- w474 stop-if-true
            n160 = Increment(x=w482) -> (x+1=w473:i32)
            n161 = Add(x=w483, y=w484) -> (x+y=w472:i32)
            n162 = Index Array(array=w486, index (row)=w473, index (col)=w472) -> (element=w481:T2)
            n163 = Multiply(x=w484, y=-1) -> (x*y=w476:i32)
            n164 = Unbundle By Name(w481) -> ("Piece.Color"=w480:T1, "Piece.Type"=w479:T4)
            n165 = Equal?(x=w476, y=2) -> (x = y?=w474:bool)
            n166 = Equal?(x=w467, y=w480) -> (x = y?=w478:bool)
            n167 = Not Equal?(x=w479, y=#typedef_PieceType."None") -> (x != y?=w477:bool)
            n168 = Build Array(w473, w472) -> (w471:i32[])
            n169 = And(x=w478, y=w477) -> (x .and. y?=w470:bool)
            n170 = Not(x=w470) -> (.not. x?=w469:bool)
          }
          n171 = while {
            tunnel: w394 -> [w466]
            tunnel: w399 -> [w462]
            tunnel: w400 -> [w463]
            shift-right: [w456] -> _
            shift-left: 2 -> [w464]
            tunnel: [w451] -> w397 mode=indexing if=w449
            tunnel: w392 -> [w447]
            stop <- w454 stop-if-true
            n172 = Decrement(x=w462) -> (x-1=w453:i32)
            n173 = Add(x=w463, y=w464) -> (x+y=w452:i32)
            n174 = Index Array(array=w466, index (row)=w453, index (col)=w452) -> (element=w461:T2)
            n175 = Multiply(x=w464, y=-1) -> (x*y=w456:i32)
            n176 = Unbundle By Name(w461) -> ("Piece.Color"=w460:T1, "Piece.Type"=w459:T4)
            n177 = Equal?(x=w456, y=2) -> (x = y?=w454:bool)
            n178 = Equal?(x=w447, y=w460) -> (x = y?=w458:bool)
            n179 = Not Equal?(x=w459, y=#typedef_PieceType."None") -> (x != y?=w457:bool)
            n180 = Build Array(w453, w452) -> (w451:i32[])
            n181 = And(x=w458, y=w457) -> (x .and. y?=w450:bool)
            n182 = Not(x=w450) -> (.not. x?=w449:bool)
          }
          n183 = while {
            tunnel: w394 -> [w426]
            tunnel: w399 -> [w413]
            tunnel: w400 -> [w411]
            shift-right: [w419] -> _
            shift-left: 2 -> [w412]
            tunnel: [w416] -> w395 mode=indexing if=w414
            tunnel: w392 -> [w407]
            stop <- w417 stop-if-true
            n184 = Add(x=w413, y=w412) -> (x+y=w410:i32)
            n185 = Decrement(x=w411) -> (x-1=w409:i32)
            n186 = Index Array(array=w426, index (row)=w410, index (col)=w409) -> (element=w424:T2)
            n187 = Multiply(x=w412, y=-1) -> (x*y=w419:i32)
            n188 = Unbundle By Name(w424) -> ("Piece.Color"=w423:T1, "Piece.Type"=w422:T4)
            n189 = Equal?(x=w419, y=2) -> (x = y?=w417:bool)
            n190 = Equal?(x=w407, y=w423) -> (x = y?=w421:bool)
            n191 = Not Equal?(x=w422, y=#typedef_PieceType."None") -> (x != y?=w420:bool)
            n192 = Build Array(w410, w409) -> (w416:i32[])
            n193 = And(x=w421, y=w420) -> (x .and. y?=w415:bool)
            n194 = Not(x=w415) -> (.not. x?=w414:bool)
          }
          n195 = Insert Into Array(array=w398, new element #1=w397, new element #2=w396, new element #3=w395) -> (w391:i32[][])  [unwired: 2 in]
        }
        frame "Bishop" {
          n196 = Index Array(array=w500, index #1=0 ("index (row)"), index #2=1 ("index")) -> (element #1=w494:i32, element #2=w493:i32)
          n197 = while {
            tunnel: w495 -> [w519]
            shift-right: [w508] -> _
            shift-left: w494 -> [w520]
            shift-right: [w505] -> _
            shift-left: w493 -> [w521]
            tunnel: [w507] -> w496 mode=indexing if=w506
            tunnel: w492 -> [w503]
            stop <- w509 stop-if-true
            n198 = Decrement(x=w520) -> (x-1=w508:i32)
            n199 = Decrement(x=w521) -> (x-1=w505:i32)
            n200 = Index Array(array=w519, index (row)=w508, index (col)=w505) -> (element=w518:T2)
            n201 = Unbundle By Name(w518) -> ("Piece.Color"=w514:T1, "Piece.Type"=w517:T4)
            n202 = Less Or Equal?(x=w508, y=0) -> (x <= y?=w511:bool)
            n203 = Less Or Equal?(x=w505, y=0) -> (x <= y?=w510:bool)
            n204 = Equal?(x=#typedef_PieceType."None", y=w517) -> (x = y?=w515:bool)
            n205 = case shown="False" w515 {
              tunnel: w514 -> [w528 _]
              tunnel: [TRUE FALSE] -> w512
              tunnel: [w523 TRUE] -> w506
              tunnel: w503 -> [w522 _]
              frame False {
                n206 = Not Equal?(x=w522, y=w528) -> (x != y?=w526:bool)
                n207 = Select(t=TRUE, s=w526, f=FALSE) -> (s? t:f=w523:bool)
              }
              frame True {
              }
            }
            n208 = Compound Arithmetic op=OR(w512, w511, w510) -> (w509:bool)
            n209 = Build Array(w508, w505) -> (w507:i32[])
          }
          n210 = while {
            tunnel: w495 -> [w547]
            shift-right: [w536] -> _
            shift-left: w494 -> [w548]
            shift-right: [w533] -> _
            shift-left: w493 -> [w549]
            tunnel: [w535] -> w497 mode=indexing if=w534
            tunnel: w492 -> [w531]
            stop <- w537 stop-if-true
            n211 = Decrement(x=w548) -> (x-1=w536:i32)
            n212 = Increment(x=w549) -> (x+1=w533:i32)
            n213 = Index Array(array=w547, index (row)=w536, index (col)=w533) -> (element=w546:T2)
            n214 = Unbundle By Name(w546) -> ("Piece.Color"=w542:T1, "Piece.Type"=w545:T4)
            n215 = Less Or Equal?(x=w536, y=0) -> (x <= y?=w539:bool)
            n216 = Greater Or Equal?(x=w533, y=7) -> (x >= y?=w538:bool)
            n217 = Equal?(x=#typedef_PieceType."None", y=w545) -> (x = y?=w543:bool)
            n218 = case shown="False" w543 {
              tunnel: w542 -> [w556 _]
              tunnel: [TRUE FALSE] -> w540
              tunnel: [w551 TRUE] -> w534
              tunnel: w531 -> [w550 _]
              frame False {
                n219 = Not Equal?(x=w550, y=w556) -> (x != y?=w554:bool)
                n220 = Select(t=TRUE, s=w554, f=FALSE) -> (s? t:f=w551:bool)
              }
              frame True {
              }
            }
            n221 = Compound Arithmetic op=OR(w540, w539, w538) -> (w537:bool)
            n222 = Build Array(w536, w533) -> (w535:i32[])
          }
          n223 = while {
            tunnel: w495 -> [w602]
            shift-right: [w592] -> _
            shift-left: w494 -> [w603]
            shift-right: [w589] -> _
            shift-left: w493 -> [w604]
            tunnel: [w591] -> w499 mode=indexing if=w590
            tunnel: w492 -> [w587]
            stop <- w593 stop-if-true
            w588 = 7 ("y")
            n224 = Increment(x=w603) -> (x+1=w592:i32)
            n225 = Increment(x=w604) -> (x+1=w589:i32)
            n226 = Index Array(array=w602, index (row)=w592, index (col)=w589) -> (element=w601:T2)
            n227 = Unbundle By Name(w601) -> ("Piece.Color"=w597:T1, "Piece.Type"=w600:T4)
            n228 = Greater Or Equal?(x=w592, y=w588) -> (x >= y?=w595:bool)
            n229 = Greater Or Equal?(x=w589, y=w588) -> (x >= y?=w594:bool)
            n230 = Equal?(x=#typedef_PieceType."None", y=w600) -> (x = y?=w598:bool)
            n231 = case shown="False" w598 {
              tunnel: w597 -> [w611 _]
              tunnel: [TRUE FALSE] -> w596
              tunnel: [w606 TRUE] -> w590
              tunnel: w587 -> [w605 _]
              frame False {
                n232 = Not Equal?(x=w605, y=w611) -> (x != y?=w609:bool)
                n233 = Select(t=TRUE, s=w609, f=FALSE) -> (s? t:f=w606:bool)
              }
              frame True {
              }
            }
            n234 = Compound Arithmetic op=OR(w596, w595, w594) -> (w593:bool)
            n235 = Build Array(w592, w589) -> (w591:i32[])
          }
          n236 = while {
            tunnel: w495 -> [w575]
            shift-right: [w564] -> _
            shift-left: w494 -> [w576]
            shift-right: [w561] -> _
            shift-left: w493 -> [w577]
            tunnel: [w563] -> w498 mode=indexing if=w562
            tunnel: w492 -> [w559]
            stop <- w565 stop-if-true
            n237 = Increment(x=w576) -> (x+1=w564:i32)
            n238 = Decrement(x=w577) -> (x-1=w561:i32)
            n239 = Index Array(array=w575, index (row)=w564, index (col)=w561) -> (element=w574:T2)
            n240 = Unbundle By Name(w574) -> ("Piece.Color"=w570:T1, "Piece.Type"=w573:T4)
            n241 = Greater Or Equal?(x=w564, y=7) -> (x >= y?=w567:bool)
            n242 = Less Or Equal?(x=w561, y=0) -> (x <= y?=w566:bool)
            n243 = Equal?(x=#typedef_PieceType."None", y=w573) -> (x = y?=w571:bool)
            n244 = case shown="False" w571 {
              tunnel: w570 -> [w584 _]
              tunnel: [TRUE FALSE] -> w568
              tunnel: [w579 TRUE] -> w562
              tunnel: w559 -> [w578 _]
              frame False {
                n245 = Not Equal?(x=w578, y=w584) -> (x != y?=w582:bool)
                n246 = Select(t=TRUE, s=w582, f=FALSE) -> (s? t:f=w579:bool)
              }
              frame True {
              }
            }
            n247 = Compound Arithmetic op=OR(w568, w567, w566) -> (w565:bool)
            n248 = Build Array(w564, w561) -> (w563:i32[])
          }
          n249 = Insert Into Array(array=w499, new element #1=w498, new element #2=w497, new element #3=w496) -> (w491:i32[][])  [unwired: 2 in]
        }
        frame "Rook" {
          n250 = Index Array(array=w627, index #1=0 ("index (row)"), index #2=1 ("index")) -> (element #1=w621:i32, element #2=w620:i32)
          n251 = while {
            tunnel: w622 -> [w644]
            shift-right: [w634] -> _
            shift-left: w620 -> [w645]
            tunnel: [w636] -> w623 mode=indexing if=w635
            tunnel: w621 -> [w632]
            tunnel: [w632] -> _
            tunnel: w619 -> [w630]
            stop <- w637 stop-if-true
            n252 = Decrement(x=w645) -> (x-1=w634:i32)
            n253 = Index Array(array=w644, index (row)=w632, index (col)=w634) -> (element=w643:T2)
            n254 = Unbundle By Name(w643) -> ("Piece.Color"=w639:T1, "Piece.Type"=w642:T4)
            n255 = Less Or Equal?(x=w634, y=0) -> (x <= y?=w631:bool)
            n256 = Equal?(x=#typedef_PieceType."None", y=w642) -> (x = y?=w640:bool)
            n257 = case shown="False" w640 {
              tunnel: w639 -> [w652 _]
              tunnel: [TRUE FALSE] -> w638
              tunnel: [w647 TRUE] -> w635
              tunnel: w630 -> [w646 _]
              frame False {
                n258 = Not Equal?(x=w646, y=w652) -> (x != y?=w650:bool)
                n259 = Select(t=TRUE, s=w650, f=FALSE) -> (s? t:f=w647:bool)
              }
              frame True {
              }
            }
            n260 = Compound Arithmetic op=OR(w638, w631) -> (w637:bool)
            n261 = Build Array(w632, w634) -> (w636:i32[])
          }
          n262 = while {
            tunnel: w622 -> [w669]
            shift-right: [w659] -> _
            shift-left: w620 -> [w670]
            tunnel: [w661] -> w624 mode=indexing if=w660
            tunnel: w621 -> [w657]
            tunnel: [w657] -> _
            tunnel: w619 -> [w655]
            stop <- w662 stop-if-true
            n263 = Increment(x=w670) -> (x+1=w659:i32)
            n264 = Index Array(array=w669, index (row)=w657, index (col)=w659) -> (element=w668:T2)
            n265 = Unbundle By Name(w668) -> ("Piece.Color"=w664:T1, "Piece.Type"=w667:T4)
            n266 = Greater Or Equal?(x=w659, y=7) -> (x >= y?=w656:bool)
            n267 = Equal?(x=#typedef_PieceType."None", y=w667) -> (x = y?=w665:bool)
            n268 = case shown="True" w665 {
              tunnel: w664 -> [w677 _]
              tunnel: [TRUE FALSE] -> w663
              tunnel: [w672 TRUE] -> w660
              tunnel: w655 -> [w671 _]
              frame False {
                n269 = Not Equal?(x=w671, y=w677) -> (x != y?=w675:bool)
                n270 = Select(t=TRUE, s=w675, f=FALSE) -> (s? t:f=w672:bool)
              }
              frame True {
              }
            }
            n271 = Compound Arithmetic op=OR(w663, w656) -> (w662:bool)
            n272 = Build Array(w657, w659) -> (w661:i32[])
          }
          n273 = while {
            tunnel: w622 -> [w719]
            shift-right: [w710] -> _
            shift-left: w621 -> [w720]
            tunnel: [w709] -> w626 mode=indexing if=w708
            tunnel: w620 -> [w706]
            tunnel: w619 -> [w705]
            stop <- w711 stop-if-true
            n274 = Increment(x=w720) -> (x+1=w710:i32)
            n275 = Index Array(array=w719, index (row)=w710, index (col)=w706) -> (element=w718:T2)
            n276 = Unbundle By Name(w718) -> ("Piece.Color"=w714:T1, "Piece.Type"=w717:T4)
            n277 = Greater Or Equal?(x=w710, y=7) -> (x >= y?=w712:bool)
            n278 = Equal?(x=#typedef_PieceType."None", y=w717) -> (x = y?=w715:bool)
            n279 = case shown="False" w715 {
              tunnel: w714 -> [w727 _]
              tunnel: [TRUE FALSE] -> w713
              tunnel: [w722 TRUE] -> w708
              tunnel: w705 -> [w721 _]
              frame False {
                n280 = Not Equal?(x=w721, y=w727) -> (x != y?=w725:bool)
                n281 = Select(t=TRUE, s=w725, f=FALSE) -> (s? t:f=w722:bool)
              }
              frame True {
              }
            }
            n282 = Compound Arithmetic op=OR(w713, w712) -> (w711:bool)
            n283 = Build Array(w710, w706) -> (w709:i32[])
          }
          n284 = while {
            tunnel: w622 -> [w694]
            shift-right: [w684] -> _
            shift-left: w621 -> [w695]
            tunnel: [w683] -> w625 mode=indexing if=w682
            tunnel: w620 -> [w681]
            tunnel: w619 -> [w680]
            stop <- w685 stop-if-true
            n285 = Decrement(x=w695) -> (x-1=w684:i32)
            n286 = Index Array(array=w694, index (row)=w684, index (col)=w681) -> (element=w693:T2)
            n287 = Unbundle By Name(w693) -> ("Piece.Color"=w689:T1, "Piece.Type"=w692:T4)
            n288 = Less Or Equal?(x=w684, y=0) -> (x <= y?=w686:bool)
            n289 = Equal?(x=#typedef_PieceType."None", y=w692) -> (x = y?=w690:bool)
            n290 = case shown="True" w690 {
              tunnel: w689 -> [w702 _]
              tunnel: [TRUE FALSE] -> w687
              tunnel: [w697 TRUE] -> w682
              tunnel: w680 -> [w696 _]
              frame False {
                n291 = Not Equal?(x=w696, y=w702) -> (x != y?=w700:bool)
                n292 = Select(t=TRUE, s=w700, f=FALSE) -> (s? t:f=w697:bool)
              }
              frame True {
              }
            }
            n293 = Compound Arithmetic op=OR(w687, w686) -> (w685:bool)
            n294 = Build Array(w684, w681) -> (w683:i32[])
          }
          n295 = Insert Into Array(array=w626, new element #1=w625, new element #2=w624, new element #3=w623) -> (w618:i32[][])  [unwired: 2 in]
        }
        frame "Queen" {
          n296 = Index Array(array=w747, index #1=0 ("index (row)"), index #2=1 ("index")) -> (element #1=w740:i32, element #2=w741:i32)
          n297 = while {
            tunnel: w742 -> [w764]
            shift-right: [w754] -> _
            shift-left: w741 -> [w765]
            tunnel: [w756] -> w735 mode=indexing if=w755
            tunnel: w740 -> [w752]
            tunnel: [w752] -> _
            tunnel: w739 -> [w750]
            stop <- w757 stop-if-true
            n298 = Decrement(x=w765) -> (x-1=w754:i32)
            n299 = Index Array(array=w764, index (row)=w752, index (col)=w754) -> (element=w763:T2)
            n300 = Unbundle By Name(w763) -> ("Piece.Color"=w759:T1, "Piece.Type"=w762:T4)
            n301 = Less Or Equal?(x=w754, y=0) -> (x <= y?=w751:bool)
            n302 = Equal?(x=#typedef_PieceType."None", y=w762) -> (x = y?=w760:bool)
            n303 = case shown="False" w760 {
              tunnel: w759 -> [w772 _]
              tunnel: [TRUE FALSE] -> w758
              tunnel: [w767 TRUE] -> w755
              tunnel: w750 -> [w766 _]
              frame False {
                n304 = Not Equal?(x=w766, y=w772) -> (x != y?=w770:bool)
                n305 = Select(t=TRUE, s=w770, f=FALSE) -> (s? t:f=w767:bool)
              }
              frame True {
              }
            }
            n306 = Compound Arithmetic op=OR(w758, w751) -> (w757:bool)
            n307 = Build Array(w752, w754) -> (w756:i32[])
          }
          n308 = while {
            tunnel: w742 -> [w789]
            shift-right: [w779] -> _
            shift-left: w741 -> [w790]
            tunnel: [w781] -> w736 mode=indexing if=w780
            tunnel: w740 -> [w777]
            tunnel: [w777] -> _
            tunnel: w739 -> [w775]
            stop <- w782 stop-if-true
            n309 = Increment(x=w790) -> (x+1=w779:i32)
            n310 = Index Array(array=w789, index (row)=w777, index (col)=w779) -> (element=w788:T2)
            n311 = Unbundle By Name(w788) -> ("Piece.Color"=w784:T1, "Piece.Type"=w787:T4)
            n312 = Greater Or Equal?(x=w779, y=7) -> (x >= y?=w776:bool)
            n313 = Equal?(x=#typedef_PieceType."None", y=w787) -> (x = y?=w785:bool)
            n314 = case shown="False" w785 {
              tunnel: w784 -> [w797 _]
              tunnel: [TRUE FALSE] -> w783
              tunnel: [w792 TRUE] -> w780
              tunnel: w775 -> [w791 _]
              frame False {
                n315 = Not Equal?(x=w791, y=w797) -> (x != y?=w795:bool)
                n316 = Select(t=TRUE, s=w795, f=FALSE) -> (s? t:f=w792:bool)
              }
              frame True {
              }
            }
            n317 = Compound Arithmetic op=OR(w783, w776) -> (w782:bool)
            n318 = Build Array(w777, w779) -> (w781:i32[])
          }
          n319 = while {
            tunnel: w742 -> [w866]
            shift-right: [w855] -> _
            shift-left: w740 -> [w867]
            shift-right: [w852] -> _
            shift-left: w741 -> [w868]
            tunnel: [w854] -> w743 mode=indexing if=w853
            tunnel: w739 -> [w850]
            stop <- w856 stop-if-true
            n320 = Decrement(x=w867) -> (x-1=w855:i32)
            n321 = Decrement(x=w868) -> (x-1=w852:i32)
            n322 = Index Array(array=w866, index (row)=w855, index (col)=w852) -> (element=w865:T2)
            n323 = Unbundle By Name(w865) -> ("Piece.Color"=w861:T1, "Piece.Type"=w864:T4)
            n324 = Less Or Equal?(x=w855, y=0) -> (x <= y?=w858:bool)
            n325 = Less Or Equal?(x=w852, y=0) -> (x <= y?=w857:bool)
            n326 = Equal?(x=#typedef_PieceType."None", y=w864) -> (x = y?=w862:bool)
            n327 = case shown="False" w862 {
              tunnel: w861 -> [w875 _]
              tunnel: [TRUE FALSE] -> w859
              tunnel: [w870 TRUE] -> w853
              tunnel: w850 -> [w869 _]
              frame False {
                n328 = Not Equal?(x=w869, y=w875) -> (x != y?=w873:bool)
                n329 = Select(t=TRUE, s=w873, f=FALSE) -> (s? t:f=w870:bool)
              }
              frame True {
              }
            }
            n330 = Compound Arithmetic op=OR(w859, w858, w857) -> (w856:bool)
            n331 = Build Array(w855, w852) -> (w854:i32[])
          }
          n332 = while {
            tunnel: w742 -> [w839]
            shift-right: [w830] -> _
            shift-left: w740 -> [w840]
            tunnel: [w829] -> w738 mode=indexing if=w828
            tunnel: w741 -> [w826]
            tunnel: w739 -> [w825]
            stop <- w831 stop-if-true
            n333 = Increment(x=w840) -> (x+1=w830:i32)
            n334 = Index Array(array=w839, index (row)=w830, index (col)=w826) -> (element=w838:T2)
            n335 = Unbundle By Name(w838) -> ("Piece.Color"=w834:T1, "Piece.Type"=w837:T4)
            n336 = Greater Or Equal?(x=w830, y=7) -> (x >= y?=w832:bool)
            n337 = Equal?(x=#typedef_PieceType."None", y=w837) -> (x = y?=w835:bool)
            n338 = case shown="False" w835 {
              tunnel: w834 -> [w847 _]
              tunnel: [TRUE FALSE] -> w833
              tunnel: [w842 TRUE] -> w828
              tunnel: w825 -> [w841 _]
              frame False {
                n339 = Not Equal?(x=w841, y=w847) -> (x != y?=w845:bool)
                n340 = Select(t=TRUE, s=w845, f=FALSE) -> (s? t:f=w842:bool)
              }
              frame True {
              }
            }
            n341 = Compound Arithmetic op=OR(w833, w832) -> (w831:bool)
            n342 = Build Array(w830, w826) -> (w829:i32[])
          }
          n343 = while {
            tunnel: w742 -> [w814]
            shift-right: [w804] -> _
            shift-left: w740 -> [w815]
            tunnel: [w803] -> w737 mode=indexing if=w802
            tunnel: w741 -> [w801]
            tunnel: w739 -> [w800]
            stop <- w805 stop-if-true
            n344 = Decrement(x=w815) -> (x-1=w804:i32)
            n345 = Index Array(array=w814, index (row)=w804, index (col)=w801) -> (element=w813:T2)
            n346 = Unbundle By Name(w813) -> ("Piece.Color"=w809:T1, "Piece.Type"=w812:T4)
            n347 = Less Or Equal?(x=w804, y=0) -> (x <= y?=w806:bool)
            n348 = Equal?(x=#typedef_PieceType."None", y=w812) -> (x = y?=w810:bool)
            n349 = case shown="False" w810 {
              tunnel: w809 -> [w822 _]
              tunnel: [TRUE FALSE] -> w807
              tunnel: [w817 TRUE] -> w802
              tunnel: w800 -> [w816 _]
              frame False {
                n350 = Not Equal?(x=w816, y=w822) -> (x != y?=w820:bool)
                n351 = Select(t=TRUE, s=w820, f=FALSE) -> (s? t:f=w817:bool)
              }
              frame True {
              }
            }
            n352 = Compound Arithmetic op=OR(w807, w806) -> (w805:bool)
            n353 = Build Array(w804, w801) -> (w803:i32[])
          }
          n354 = while {
            tunnel: w742 -> [w894]
            shift-right: [w883] -> _
            shift-left: w740 -> [w895]
            shift-right: [w880] -> _
            shift-left: w741 -> [w896]
            tunnel: [w882] -> w744 mode=indexing if=w881
            tunnel: w739 -> [w878]
            stop <- w884 stop-if-true
            n355 = Decrement(x=w895) -> (x-1=w883:i32)
            n356 = Increment(x=w896) -> (x+1=w880:i32)
            n357 = Index Array(array=w894, index (row)=w883, index (col)=w880) -> (element=w893:T2)
            n358 = Unbundle By Name(w893) -> ("Piece.Color"=w889:T1, "Piece.Type"=w892:T4)
            n359 = Less Or Equal?(x=w883, y=0) -> (x <= y?=w886:bool)
            n360 = Greater Or Equal?(x=w880, y=7) -> (x >= y?=w885:bool)
            n361 = Equal?(x=#typedef_PieceType."None", y=w892) -> (x = y?=w890:bool)
            n362 = case shown="False" w890 {
              tunnel: w889 -> [w903 _]
              tunnel: [TRUE FALSE] -> w887
              tunnel: [w898 TRUE] -> w881
              tunnel: w878 -> [w897 _]
              frame False {
                n363 = Not Equal?(x=w897, y=w903) -> (x != y?=w901:bool)
                n364 = Select(t=TRUE, s=w901, f=FALSE) -> (s? t:f=w898:bool)
              }
              frame True {
              }
            }
            n365 = Compound Arithmetic op=OR(w887, w886, w885) -> (w884:bool)
            n366 = Build Array(w883, w880) -> (w882:i32[])
          }
          n367 = while {
            tunnel: w742 -> [w949]
            shift-right: [w939] -> _
            shift-left: w740 -> [w950]
            shift-right: [w936] -> _
            shift-left: w741 -> [w951]
            tunnel: [w938] -> w746 mode=indexing if=w937
            tunnel: w739 -> [w934]
            stop <- w940 stop-if-true
            w935 = 7 ("y")
            n368 = Increment(x=w950) -> (x+1=w939:i32)
            n369 = Increment(x=w951) -> (x+1=w936:i32)
            n370 = Index Array(array=w949, index (row)=w939, index (col)=w936) -> (element=w948:T2)
            n371 = Unbundle By Name(w948) -> ("Piece.Color"=w944:T1, "Piece.Type"=w947:T4)
            n372 = Greater Or Equal?(x=w939, y=w935) -> (x >= y?=w942:bool)
            n373 = Greater Or Equal?(x=w936, y=w935) -> (x >= y?=w941:bool)
            n374 = Equal?(x=#typedef_PieceType."None", y=w947) -> (x = y?=w945:bool)
            n375 = case shown="False" w945 {
              tunnel: w944 -> [w958 _]
              tunnel: [TRUE FALSE] -> w943
              tunnel: [w953 TRUE] -> w937
              tunnel: w934 -> [w952 _]
              frame False {
                n376 = Not Equal?(x=w952, y=w958) -> (x != y?=w956:bool)
                n377 = Select(t=TRUE, s=w956, f=FALSE) -> (s? t:f=w953:bool)
              }
              frame True {
              }
            }
            n378 = Compound Arithmetic op=OR(w943, w942, w941) -> (w940:bool)
            n379 = Build Array(w939, w936) -> (w938:i32[])
          }
          n380 = while {
            tunnel: w742 -> [w922]
            shift-right: [w911] -> _
            shift-left: w740 -> [w923]
            shift-right: [w908] -> _
            shift-left: w741 -> [w924]
            tunnel: [w910] -> w745 mode=indexing if=w909
            tunnel: w739 -> [w906]
            stop <- w912 stop-if-true
            n381 = Increment(x=w923) -> (x+1=w911:i32)
            n382 = Decrement(x=w924) -> (x-1=w908:i32)
            n383 = Index Array(array=w922, index (row)=w911, index (col)=w908) -> (element=w921:T2)
            n384 = Unbundle By Name(w921) -> ("Piece.Color"=w917:T1, "Piece.Type"=w920:T4)
            n385 = Greater Or Equal?(x=w911, y=7) -> (x >= y?=w914:bool)
            n386 = Less Or Equal?(x=w908, y=0) -> (x <= y?=w913:bool)
            n387 = Equal?(x=#typedef_PieceType."None", y=w920) -> (x = y?=w918:bool)
            n388 = case shown="False" w918 {
              tunnel: w917 -> [w931 _]
              tunnel: [TRUE FALSE] -> w915
              tunnel: [w926 TRUE] -> w909
              tunnel: w906 -> [w925 _]
              frame False {
                n389 = Not Equal?(x=w925, y=w931) -> (x != y?=w929:bool)
                n390 = Select(t=TRUE, s=w929, f=FALSE) -> (s? t:f=w926:bool)
              }
              frame True {
              }
            }
            n391 = Compound Arithmetic op=OR(w915, w914, w913) -> (w912:bool)
            n392 = Build Array(w911, w908) -> (w910:i32[])
          }
          n393 = Insert Into Array(array=w746, new element #1=w745, new element #2=w744, new element #3=w743, new element #4=w738, new element #5=w737, new element #6=w736, new element #7=w735) -> (w734:i32[][])  [unwired: 2 in]
        }
        frame "King" {
          n394 = Index Array(array=w980, index #1=0 ("index (row)"), index #2=1 ("index")) -> (element #1=w964:i32, element #2=w965:i32)
          n395 = while {
            tunnel: w969 -> [w1076]
            shift-right: [w1066] -> _
            shift-left: w965 -> [w1077]
            tunnel: [w1068] -> w973 mode=indexing if=w1067
            tunnel: w964 -> [w1065]
            tunnel: [w1065] -> _
            tunnel: w968 -> [w1064]
            stop <- w1069 stop-if-true
            n396 = Decrement(x=w1077) -> (x-1=w1066:i32)
            n397 = Index Array(array=w1076, index (row)=w1065, index (col)=w1066) -> (element=w1075:T2)
            n398 = Unbundle By Name(w1075) -> ("Piece.Color"=w1071:T1, "Piece.Type"=w1074:T4)
            n399 = Equal?(x=#typedef_PieceType."None", y=w1074) -> (x = y?=w1072:bool)
            n400 = case shown="False" w1072 {
              tunnel: w1071 -> [w1084 _]
              tunnel: [TRUE FALSE] -> w1070
              tunnel: [w1079 TRUE] -> w1067
              tunnel: w1064 -> [w1078 _]
              frame False {
                n401 = Not Equal?(x=w1078, y=w1084) -> (x != y?=w1082:bool)
                n402 = Select(t=TRUE, s=w1082, f=FALSE) -> (s? t:f=w1079:bool)
              }
              frame True {
              }
            }
            n403 = Compound Arithmetic op=OR(w1070, TRUE ("value")) -> (w1069:bool)
            n404 = Build Array(w1065, w1066) -> (w1068:i32[])
          }
          n405 = while {
            tunnel: w969 -> [w1047]
            tunnel: w964 -> [w1029]
            tunnel: w965 -> [w1045]
            tunnel: w968 -> [w1048]
            tunnel: [w1027] -> w967 mode=indexing if=w1026
            stop <- TRUE stop-if-true
            n406 = Increment(x=w1045) -> (x+1=w1044:i32)
            n407 = Increment(x=w1044) -> (x+1=w1028:i32)
            n408 = Increment(x=w1028) -> (x+1=w1043:i32)
            n409 = Index Array(array=w1047, index (row)=w1029, index (col)=w1045) -> (element=w1062:T2)
            n410 = Index Array(array=w1047, index (row)=w1029, index (col)=w1028) -> (element=w1059:T2)
            n411 = Index Array(array=w1047, index (row)=w1029, index (col)=w1043) -> (element=w1060:T2)
            n412 = Index Array(array=w1047, index (row)=w1029, index (col)=w1044) -> (element=w1061:T2)
            n413 = call "AttackedSquares.vi"("Turn"=w1048, "Input Squares"=w1047) -> ("Attacked Squares"=w1046:bool[][])  [unwired: 9 in]
            n414 = Unbundle By Name(w1059) -> ("Piece.Type"=w1054:T4)
            n415 = Unbundle By Name(w1060) -> ("Piece.Type"=w1052:T4, "Piece.Moved?"=w1050:bool)
            n416 = Unbundle By Name(w1062) -> ("Piece.Moved?"=w1057:bool)
            n417 = Unbundle By Name(w1061) -> ("Piece.Type"=w1056:T4)
            n418 = Index Array(array=w1046, index (row) #1=w1029, index (col) #1=w1045, index (row) #2=w1029, index (col) #2=w1044, index (row) #3=w1029, index (col) #3=w1028, index (row) #4=w1029, index (col) #4=w1043) -> (element #1=w1042:bool, element #2=w1041:bool, element #3=w1040:bool, element #4=w1039:bool)
            n419 = Compound Arithmetic op=OR(w1042, w1041, w1040, w1039) -> (w1038:bool)
            n420 = Equal?(x=FALSE, y=w1057) -> (x = y?=w1035:bool)
            n421 = Equal?(x=#typedef_PieceType."None", y=w1056) -> (x = y?=w1034:bool)
            n422 = Equal?(x=#typedef_PieceType."None", y=w1054) -> (x = y?=w1033:bool)
            n423 = Equal?(x=#typedef_PieceType."Rook", y=w1052) -> (x = y?=w1032:bool)
            n424 = Equal?(x=w1050, y=FALSE) -> (x = y?=w1031:bool)
            n425 = Equal?(x=FALSE, y=w1038) -> (x = y?=w1030:bool)
            n426 = Compound Arithmetic op=AND(w1035, w1034, w1033, w1032, w1031, w1030) -> (w1026:bool)
            n427 = Build Array(w1029, w1028) -> (w1027:i32[])
          }
          n428 = while {
            tunnel: w969 -> [w1100]
            shift-right: [w1090] -> _
            shift-left: w965 -> [w1101]
            tunnel: [w1092] -> w974 mode=indexing if=w1091
            tunnel: w964 -> [w1089]
            tunnel: [w1089] -> _
            tunnel: w968 -> [w1088]
            stop <- w1093 stop-if-true
            n429 = Increment(x=w1101) -> (x+1=w1090:i32)
            n430 = Index Array(array=w1100, index (row)=w1089, index (col)=w1090) -> (element=w1099:T2)
            n431 = Unbundle By Name(w1099) -> ("Piece.Color"=w1095:T1, "Piece.Type"=w1098:T4)
            n432 = Equal?(x=#typedef_PieceType."None", y=w1098) -> (x = y?=w1096:bool)
            n433 = case shown="True" w1096 {
              tunnel: w1095 -> [w1108 _]
              tunnel: [TRUE FALSE] -> w1094
              tunnel: [w1103 TRUE] -> w1091
              tunnel: w1088 -> [w1102 _]
              frame False {
                n434 = Not Equal?(x=w1102, y=w1108) -> (x != y?=w1106:bool)
                n435 = Select(t=TRUE, s=w1106, f=FALSE) -> (s? t:f=w1103:bool)
              }
              frame True {
              }
            }
            n436 = Compound Arithmetic op=OR(w1094, TRUE ("value")) -> (w1093:bool)
            n437 = Build Array(w1089, w1090) -> (w1092:i32[])
          }
          n438 = while {
            tunnel: w969 -> [w1172]
            shift-right: [w1164] -> _
            shift-left: w964 -> [w1173]
            shift-right: [w1161] -> _
            shift-left: w965 -> [w1174]
            tunnel: [w1163] -> w977 mode=indexing if=w1162
            tunnel: w968 -> [w1160]
            stop <- w1165 stop-if-true
            n439 = Decrement(x=w1173) -> (x-1=w1164:i32)
            n440 = Decrement(x=w1174) -> (x-1=w1161:i32)
            n441 = Index Array(array=w1172, index (row)=w1164, index (col)=w1161) -> (element=w1171:T2)
            n442 = Unbundle By Name(w1171) -> ("Piece.Color"=w1167:T1, "Piece.Type"=w1170:T4)
            n443 = Equal?(x=#typedef_PieceType."None", y=w1170) -> (x = y?=w1168:bool)
            n444 = case shown="True" w1168 {
              tunnel: w1167 -> [w1181 _]
              tunnel: [TRUE FALSE] -> w1166
              tunnel: [w1176 TRUE] -> w1162
              tunnel: w1160 -> [w1175 _]
              frame False {
                n445 = Not Equal?(x=w1175, y=w1181) -> (x != y?=w1179:bool)
                n446 = Select(t=TRUE, s=w1179, f=FALSE) -> (s? t:f=w1176:bool)
              }
              frame True {
              }
            }
            n447 = Compound Arithmetic op=OR(w1166, TRUE ("value")) -> (w1165:bool)
            n448 = Build Array(w1164, w1161) -> (w1163:i32[])
          }
          n449 = while {
            tunnel: w969 -> [w1148]
            shift-right: [w1140] -> _
            shift-left: w964 -> [w1149]
            tunnel: [w1139] -> w976 mode=indexing if=w1138
            tunnel: w965 -> [w1137]
            tunnel: w968 -> [w1136]
            stop <- w1141 stop-if-true
            n450 = Increment(x=w1149) -> (x+1=w1140:i32)
            n451 = Index Array(array=w1148, index (row)=w1140, index (col)=w1137) -> (element=w1147:T2)
            n452 = Unbundle By Name(w1147) -> ("Piece.Color"=w1143:T1, "Piece.Type"=w1146:T4)
            n453 = Equal?(x=#typedef_PieceType."None", y=w1146) -> (x = y?=w1144:bool)
            n454 = case shown="False" w1144 {
              tunnel: w1143 -> [w1156 _]
              tunnel: [TRUE FALSE] -> w1142
              tunnel: [w1151 TRUE] -> w1138
              tunnel: w1136 -> [w1150 _]
              frame False {
                n455 = Not Equal?(x=w1150, y=w1156) -> (x != y?=w1154:bool)
                n456 = Select(t=TRUE, s=w1154, f=FALSE) -> (s? t:f=w1151:bool)
              }
              frame True {
              }
            }
            n457 = Compound Arithmetic op=OR(w1142, TRUE ("value")) -> (w1141:bool)
            n458 = Build Array(w1140, w1137) -> (w1139:i32[])
          }
          n459 = while {
            tunnel: w969 -> [w1124]
            shift-right: [w1116] -> _
            shift-left: w964 -> [w1125]
            tunnel: [w1115] -> w975 mode=indexing if=w1114
            tunnel: w965 -> [w1113]
            tunnel: w968 -> [w1112]
            stop <- w1117 stop-if-true
            n460 = Decrement(x=w1125) -> (x-1=w1116:i32)
            n461 = Index Array(array=w1124, index (row)=w1116, index (col)=w1113) -> (element=w1123:T2)
            n462 = Unbundle By Name(w1123) -> ("Piece.Color"=w1119:T1, "Piece.Type"=w1122:T4)
            n463 = Equal?(x=#typedef_PieceType."None", y=w1122) -> (x = y?=w1120:bool)
            n464 = case shown="True" w1120 {
              tunnel: w1119 -> [w1132 _]
              tunnel: [TRUE FALSE] -> w1118
              tunnel: [w1127 TRUE] -> w1114
              tunnel: w1112 -> [w1126 _]
              frame False {
                n465 = Not Equal?(x=w1126, y=w1132) -> (x != y?=w1130:bool)
                n466 = Select(t=TRUE, s=w1130, f=FALSE) -> (s? t:f=w1127:bool)
              }
              frame True {
              }
            }
            n467 = Compound Arithmetic op=OR(w1118, TRUE ("value")) -> (w1117:bool)
            n468 = Build Array(w1116, w1113) -> (w1115:i32[])
          }
          n469 = while {
            tunnel: w969 -> [w996]
            tunnel: w964 -> [w994]
            tunnel: w965 -> [w1012]
            tunnel: w968 -> [w983]
            tunnel: [w998] -> w966 mode=indexing if=w997
            stop <- TRUE stop-if-true
            n470 = Decrement(x=w1012) -> (x-1=w1011:i32)
            n471 = Decrement(x=w1011) -> (x-1=w999:i32)
            n472 = Decrement(x=w999) -> (x-1=w995:i32)
            n473 = Decrement(x=w995) -> (x-1=w993:i32)
            n474 = call "AttackedSquares.vi"("Turn"=w983, "Input Squares"=w996) -> ("Attacked Squares"=w1013:bool[][])  [unwired: 9 in]
            n475 = Index Array(array=w996, index (row)=w994, index (col)=w1012) -> (element=w1025:T2)
            n476 = Index Array(array=w996, index (row)=w994, index (col)=w999) -> (element=w1022:T2)
            n477 = Index Array(array=w996, index (row)=w994, index (col)=w995) -> (element=w1023:T2)
            n478 = Index Array(array=w996, index (row)=w994, index (col)=w993) -> (element=w991:T2)
            n479 = Index Array(array=w996, index (row)=w994, index (col)=w1011) -> (element=w1024:T2)
            n480 = Unbundle By Name(w1022) -> ("Piece.Type"=w1017:T4)
            n481 = Unbundle By Name(w1025) -> ("Piece.Moved?"=w1020:bool)
            n482 = Unbundle By Name(w1024) -> ("Piece.Type"=w1019:T4)
            n483 = Unbundle By Name(w991) -> ("Piece.Type"=w990:T4, "Piece.Moved?"=w988:bool)
            n484 = Unbundle By Name(w1023) -> ("Piece.Type"=w1015:T4)
            n485 = Index Array(array=w1013, index (row) #1=w994, index (col) #1=w1012, index (row) #2=w994, index (col) #2=w1011, index (row) #3=w994, index (col) #3=w999, index (row) #4=w994, index (col) #4=w995, index (row) #5=w994, index (col) #5=w993) -> (element #1=w1010:bool, element #2=w1009:bool, element #3=w1008:bool, element #4=w1007:bool, element #5=w992:bool)
            n486 = Compound Arithmetic op=OR(w1010, w1009, w1008, w1007, w992) -> (w1006:bool)
            n487 = Equal?(x=FALSE, y=w1020) -> (x = y?=w1003:bool)
            n488 = Equal?(x=#typedef_PieceType."None", y=w1019) -> (x = y?=w1002:bool)
            n489 = Equal?(x=#typedef_PieceType."Rook", y=w990) -> (x = y?=w986:bool)
            n490 = Equal?(x=#typedef_PieceType."None", y=w1017) -> (x = y?=w1001:bool)
            n491 = Equal?(x=w988, y=FALSE) -> (x = y?=w985:bool)
            n492 = Equal?(x=#typedef_PieceType."None", y=w1015) -> (x = y?=w1000:bool)
            n493 = Equal?(x=FALSE, y=w1006) -> (x = y?=w984:bool)
            n494 = Compound Arithmetic op=AND(w1003, w1002, w1001, w1000, w986, w985, w984) -> (w997:bool)
            n495 = Build Array(w994, w999) -> (w998:i32[])
          }
          n496 = while {
            tunnel: w969 -> [w1197]
            shift-right: [w1189] -> _
            shift-left: w964 -> [w1198]
            shift-right: [w1186] -> _
            shift-left: w965 -> [w1199]
            tunnel: [w1188] -> w978 mode=indexing if=w1187
            tunnel: w968 -> [w1185]
            stop <- w1190 stop-if-true
            n497 = Decrement(x=w1198) -> (x-1=w1189:i32)
            n498 = Increment(x=w1199) -> (x+1=w1186:i32)
            n499 = Index Array(array=w1197, index (row)=w1189, index (col)=w1186) -> (element=w1196:T2)
            n500 = Unbundle By Name(w1196) -> ("Piece.Color"=w1192:T1, "Piece.Type"=w1195:T4)
            n501 = Equal?(x=#typedef_PieceType."None", y=w1195) -> (x = y?=w1193:bool)
            n502 = case shown="True" w1193 {
              tunnel: w1192 -> [w1206 _]
              tunnel: [TRUE FALSE] -> w1191
              tunnel: [w1201 TRUE] -> w1187
              tunnel: w1185 -> [w1200 _]
              frame False {
                n503 = Not Equal?(x=w1200, y=w1206) -> (x != y?=w1204:bool)
                n504 = Select(t=TRUE, s=w1204, f=FALSE) -> (s? t:f=w1201:bool)
              }
              frame True {
              }
            }
            n505 = Compound Arithmetic op=OR(w1191, TRUE ("value")) -> (w1190:bool)
            n506 = Build Array(w1189, w1186) -> (w1188:i32[])
          }
          n507 = while {
            tunnel: w969 -> [w1247]
            shift-right: [w1239] -> _
            shift-left: w964 -> [w1248]
            shift-right: [w1236] -> _
            shift-left: w965 -> [w1249]
            tunnel: [w1238] -> w961 mode=indexing if=w1237
            tunnel: w968 -> [w1235]
            stop <- w1240 stop-if-true
            n508 = Increment(x=w1248) -> (x+1=w1239:i32)
            n509 = Increment(x=w1249) -> (x+1=w1236:i32)
            n510 = Index Array(array=w1247, index (row)=w1239, index (col)=w1236) -> (element=w1246:T2)
            n511 = Unbundle By Name(w1246) -> ("Piece.Color"=w1242:T1, "Piece.Type"=w1245:T4)
            n512 = Equal?(x=#typedef_PieceType."None", y=w1245) -> (x = y?=w1243:bool)
            n513 = case shown="False" w1243 {
              tunnel: w1242 -> [w1256 _]
              tunnel: [TRUE FALSE] -> w1241
              tunnel: [w1251 TRUE] -> w1237
              tunnel: w1235 -> [w1250 _]
              frame False {
                n514 = Not Equal?(x=w1250, y=w1256) -> (x != y?=w1254:bool)
                n515 = Select(t=TRUE, s=w1254, f=FALSE) -> (s? t:f=w1251:bool)
              }
              frame True {
              }
            }
            n516 = Compound Arithmetic op=OR(w1241, TRUE ("value")) -> (w1240:bool)
            n517 = Build Array(w1239, w1236) -> (w1238:i32[])
          }
          n518 = while {
            tunnel: w969 -> [w1222]
            shift-right: [w1214] -> _
            shift-left: w964 -> [w1223]
            shift-right: [w1211] -> _
            shift-left: w965 -> [w1224]
            tunnel: [w1213] -> w979 mode=indexing if=w1212
            tunnel: w968 -> [w1210]
            stop <- w1215 stop-if-true
            n519 = Increment(x=w1223) -> (x+1=w1214:i32)
            n520 = Decrement(x=w1224) -> (x-1=w1211:i32)
            n521 = Index Array(array=w1222, index (row)=w1214, index (col)=w1211) -> (element=w1221:T2)
            n522 = Unbundle By Name(w1221) -> ("Piece.Color"=w1217:T1, "Piece.Type"=w1220:T4)
            n523 = Equal?(x=#typedef_PieceType."None", y=w1220) -> (x = y?=w1218:bool)
            n524 = case shown="False" w1218 {
              tunnel: w1217 -> [w1231 _]
              tunnel: [TRUE FALSE] -> w1216
              tunnel: [w1226 TRUE] -> w1212
              tunnel: w1210 -> [w1225 _]
              frame False {
                n525 = Not Equal?(x=w1225, y=w1231) -> (x != y?=w1229:bool)
                n526 = Select(t=TRUE, s=w1229, f=FALSE) -> (s? t:f=w1226:bool)
              }
              frame True {
              }
            }
            n527 = Compound Arithmetic op=OR(w1216, TRUE ("value")) -> (w1215:bool)
            n528 = Build Array(w1214, w1211) -> (w1213:i32[])
          }
          n529 = Insert Into Array(array=w961, new element #1=w979, new element #2=w978, new element #3=w977, new element #4=w976, new element #5=w975, new element #6=w974, new element #7=w973, new element #8=w967, new element #9=w966) -> (w972:i32[][])  [unwired: 2 in]
          n530 = call "InRangePosition.vi"("Input Positions in"=w967) -> ("Output Positions"=w963:i32[][])  [unwired: 10 in]
          n531 = call "InRangePosition.vi"("Input Positions in"=w966) -> ("Output Positions"=w962:i32[][])  [unwired: 10 in]
        }
      }
      n532 = Equal?(x=w58, y=i32[][] [[-1]]) -> (x = y?=w60:bool[][])
      n533 = Equal?(x=w45, y=i32[][] [[-1]]) -> (x = y?=w48:bool[][])
      n534 = Equal?(x=w54, y=i32[][] [[-1]]) -> (x = y?=w56:bool[][])
      n535 = Equal?(x=w49, y=i32[][] [[-1]]) -> (x = y?=w52:bool[][])
      n536 = Or Array Elements(Boolean array=w60) -> (logical OR=w59:bool)
      n537 = Or Array Elements(Boolean array=w48) -> (logical OR=w46:bool)
      n538 = Or Array Elements(Boolean array=w56) -> (logical OR=w53:bool)
      n539 = Initialize Array(FALSE, w62, w62) -> (w44:bool[][])
      n540 = Or Array Elements(Boolean array=w52) -> (logical OR=w50:bool)
      n541 = case shown="True" w59 {
        tunnel: w44 -> [w104 w107]
        tunnel: w58 -> [_ w106]
        tunnel: [w104 w105] -> w39
        frame True {
        }
        frame False {
          n542 = for {
            tunnel: w106 -> [w114] mode=indexing
            shift-right: [w108] -> w105
            shift-left: w107 -> [w115]
            n543 = Index Array(array=w114, index #1=0 ("index"), index #2=1 ("index")) -> (element #1=w111:i32, element #2=w110:i32)
            n544 = Replace Array Subset(array=w115, new element=TRUE ("new element/subarray"), index (row)=w111, index (col)=w110) -> (w108:bool[][])
          }
        }
      }
      "Last Square" <- w39
      n545 = case shown="False" w46 {
        tunnel: w44 -> [w68 w71]
        tunnel: w45 -> [_ w70]
        tunnel: [w68 w69] -> w33
        frame True {
        }
        frame False {
          n546 = for {
            tunnel: w70 -> [w78] mode=indexing
            shift-right: [w72] -> w69
            shift-left: w71 -> [w79]
            n547 = Index Array(array=w78, index #1=0 ("index"), index #2=1 ("index")) -> (element #1=w75:i32, element #2=w74:i32)
            n548 = Replace Array Subset(array=w79, new element=TRUE ("new element/subarray"), index (row)=w75, index (col)=w74) -> (w72:bool[][])
          }
        }
      }
      "Long Castle" <- w33
      n549 = case shown="True" w53 {
        tunnel: w44 -> [w92 w95]
        tunnel: w54 -> [_ w94]
        tunnel: [w92 w93] -> w37
        frame True {
        }
        frame False {
          n550 = for {
            tunnel: w94 -> [w102] mode=indexing
            shift-right: [w96] -> w93
            shift-left: w95 -> [w103]
            n551 = Index Array(array=w102, index #1=0 ("index"), index #2=1 ("index")) -> (element #1=w99:i32, element #2=w98:i32)
            n552 = Replace Array Subset(array=w103, new element=TRUE ("new element/subarray"), index (row)=w99, index (col)=w98) -> (w96:bool[][])
          }
        }
      }
      "Beat in the Passage" <- w37
      n553 = case shown="False" w50 {
        tunnel: w44 -> [w80 w83]
        tunnel: w49 -> [_ w82]
        tunnel: [w80 w81] -> w35
        frame True {
        }
        frame False {
          n554 = for {
            tunnel: w82 -> [w90] mode=indexing
            shift-right: [w84] -> w81
            shift-left: w83 -> [w91]
            n555 = Index Array(array=w90, index #1=0 ("index"), index #2=1 ("index")) -> (element #1=w87:i32, element #2=w86:i32)
            n556 = Replace Array Subset(array=w91, new element=TRUE ("new element/subarray"), index (row)=w87, index (col)=w86) -> (w84:bool[][])
          }
        }
      }
      "Short Castle" <- w35
      n557 = call "InRangePosition.vi"("Input Positions in"=w63) -> ("Output Positions"=w32:i32[][])  [unwired: 10 in]
      n558 = Index Array(array=w41, index #1=0 ("index"), index #2=1 ("index")) -> (element #1=w30:i32, element #2=w31:i32)
      n559 = Index Array(array=w39, index (row)=w30, index (col)=w31) -> (element=→"Last Square?":bool)
      n560 = Index Array(array=w37, index (row)=w30, index (col)=w31) -> (element=→"Beat in the Passage?":bool)
      n561 = Index Array(array=w33, index (row)=w30, index (col)=w31) -> (element=→"Long Castle?":bool)
      n562 = Index Array(array=w35, index (row)=w30, index (col)=w31) -> (element=→"Short Castle?":bool)
    }
  }
  n563 = call "CreateBoard.vi"("Squares type"="Input Squares") -> ("Board"=→"?":u16[][])  [unwired: 10 in]
  n564 = Equal?(x=w16, y=i32[][] []) -> (x = y?=w18:bool[][])
  n565 = Or Array Elements(Boolean array=w18) -> (logical OR=w17:bool)
  n566 = Initialize Array(FALSE, w15, w15) -> (w13:bool[][])
  n567 = case shown="False" w17 {
    tunnel: w13 -> [w1259 w1262]
    tunnel: w16 -> [_ w1261]
    tunnel: [w1259 w1260] -> w12
    frame True {
    }
    frame False {
      n568 = for {
        tunnel: w1261 -> [w1269] mode=indexing
        shift-right: [w1263] -> w1260
        shift-left: w1262 -> [w1270]
        n569 = Index Array(array=w1269, index #1=0 ("index"), index #2=1 ("index")) -> (element #1=w1266:i32, element #2=w1265:i32)
        n570 = Replace Array Subset(array=w1270, new element=TRUE ("new element/subarray"), index (row)=w1266, index (col)=w1265) -> (w1263:bool[][])
      }
    }
  }
  "Possible Moves" <- w12
  n571 = Index Array(array="Move to", index #1=0 ("index"), index #2=1 ("index")) -> (element #1=w9:i32, element #2=w8:i32)
  n572 = Index Array(array=w12, index (row)=w9, index (col)=w8) -> (element=→"Possible Move?":bool)
